vi "main.vi"() -> ()   [LabVIEW 2019]
uses:
  SubVI/ctl/335 state.ctl
  SubVI/ctl/Instrument Type.ctl
  SubVI/ctl/9T mag field stauts.ctl
  SubVI/ctl/warning.ctl
  SubVI/ctl/Gating type.ctl
  SubVI/ctl/Instrument.ctl
  <vilib>/NI/Modbus Library/API/Master/Modbus Master.lvclass
  SubVI/ctl/limit.ctl
  SubVI/ctl/set type.ctl
  SubVI/ctl/config.ctl
  SubVI/ctl/initialize.ctl
  <vilib>/NI/Modbus Library/API/Wrapper/Create TCP Master.vi
  lib/QDInstrument.dll
  SubVI/SubVI.lvlib
  SubVI/Add Seq.lvlib
  SubVI/User lib.lvlib
  <vilib>/NI/Modbus Library/API/Wrapper/API Main.lvlib
  SubVI/Get value.lvlib
  lib/Lake Shore 335/Lake Shore 335.lvlib
  SubVI/9T cmag.lvlib
  SubVI/nematic.lvlib
  lib/Lake Shore 325/Lake Shore 325.lvlib
  lib/Lake Shore 340/Lake Shore Cryotronics 340.lvlib
  SubVI/initialize.lvlib
panel:
  in  "gating type":T1
  out "?":string
  in  "行数":i32
  in  "是否处理":bool[](array[boolean])
  in  "层数":i32
  out "pzt volt":i32
  in  "warning":T2
  in  "Instrument Type":T3=enum."lengtou2"
  out "数据文件":path
  out "Aborting":bool
  in  "选项卡控件":T4(tab)=enum."335 2"
  out "Field":dbl
  out "Temperature":dbl
  in  "?":T5={"Field"=0.0, "Rate "=100.0, "Mode"=0, "Approach"=0, "field set"=FALSE} {"Approach" items=["Linear", "NoOvershoot", "Oscillate"]; "Mode" items=["Persistent", "Driven"]; "Rate" min=0.0 max=100.0; "Field" min=-140000.0 max=140000.0}
  in  "?":T6={"Temperature"=300.0, "Rate"=10.0, "Mode"=0, "temp set"=FALSE} {"Mode" items=["FastSettle", "NoOvershoot"]; "Rate" min=0.0 max=10.0; "Temperature" min=2.0 max=400.0}
  out "Status":i32(ring) items=["TemperatureUnknown"=0, "Stable"=1, "Tracking"=2, "Near"=5, "Chasing"=6, "Filling"=7, "Standby"=10, "Disabled"=13, "ImpedanceNotFunction"=14, "TempFailure"=15]
  out "Field Status":i32(ring) items=["MagnetUnknown"=0, "StablePersistent"=1, "WarmingSwitch"=2, "CoolingSwitch"=3, "StableDriven"=4, "Iterating"=5, "Charging"=6, "Discharging"=7, "CurrentError"=8, "MagnetFailure"=15]
  out "Chamber Status":i32(ring) items=["ChamberUnknown"=0, "PurgedAndSealed"=1, "VentedAndSealed"=2, "Sealed"=3, "Purging"=4, "Venting"=5, "PreHiVac"=6, "HighVac"=7, "PumpContinuous"=8, "VentContinuous"=9, "ChamberFailure"=15]
  in  "?":cluster{"chamber set":bool, "Code":i32} {"Code" items=["Seal", "PurgeAndSeal", "VentAndSeal", "PumpContinuous", "VentContinuous", "HighVacuum"]}
  out "Position":dbl
  in  "?":T7 {"Mode" items=["MoveToPosition", "MoveToLimitAndDefinePosition", "DefinePosition"]; "Speed" max=10}
  out "Rotate Temp":dbl
  in  "?":T8={"Temperature"=300.0, "Rate"=10.0, "temp set"=FALSE} {"Rate" min=0.0 max=10.0; "Temperature" min=2.0 max=400.0}
  in  "压缩机开启":bool
  in  "压缩机自动停机":bool=TRUE
  in  "自动控制":bool=TRUE
  out "325 Temp":dbl
  out "簇 2":T10 {"Heater Range" items=["Off", "Low (On)", "Medium", "High"]; "Heater Range 2" items=["Off", "Low (On)", "Medium", "High"]; "335 Status" items=["Unknow", "Stable", "Following Warm", "Following Cold", "Unfollowing"]}
  out "Out-plane angle":dbl
  in  "Position":T11
  in  "?":T12={"Field(Oe)"=0.0, "Approach"=enum."Linear", "Set Field"=FALSE, "Rate(Oe/s） "=30.0} {"Rate(Oe/s）" min=0.0 max=500.0; "Field(Oe)" min=-11000.0 max=11000.0}
  out "Field (Oe)":dbl
  out "Field Status":T13=enum."Stable"
  in  "335 2":T14={"Temperature"=300.0, "Rate (K/min)"=1.0, "Set Temp"=FALSE} {"Rate (K/min)" min=0.0 max=3.0; "Temperature" min=2.0 max=350.0}
  in  "压缩机启停":bool
  out "前面板":T15 {"340-A Status" items=["Unknow", "Stable", "Following Warm", "Following Cold", "Unfollowing"]; "Heater Range" items=["Off", "Low (On)", "High"]; "Heater Range 2" items=["Off", "Level 1", "Level 2", "Level 3", "Level 4", "Level 5"]; "340-B Status" items=["Unknow", "Stable", "Following Warm", "Following Cold", "Unfollowing"]}
  out "In-plane":dbl
  out "Out-plane":dbl
  in  "position":T16
  in  "?":T17={"Field(Oe)"=0.0, "Approach"=enum."Linear", "Field set"=FALSE, "Rate "=100.0} {"Rate" min=0.0 max=100.0; "Field(Oe)" min=-90000.0 max=90000.0}
  in  "?":T18={"Temperature"=300.0, "Rate"=10.0, "Temp set"=FALSE, "Ctrl On"=FALSE} {"Rate" min=0.0 max=10.0; "Temperature" min=2.0 max=400.0}
  in  "?":cluster{"Chamber set":bool, "Code":i32} {"Code" items=["Seal", "PurgeAndSeal", "VentAndSeal", "PumpContinuous", "VentContinuous", "HighVacuum"]}
  out "?":T19 {"Loop1 Output (%)" format="%.2f"; "Loop2 Output (%)" format="%.2f"}
  out "Temperature":dbl
  out "Temp Status":T9 items=["Unknow", "Stable", "Following Warm", "Following Cold", "Unfollowing"]
  out "Field (Oe)":dbl
  out "Field status":T13=enum."Stable"
  out "oscillating":bool=TRUE
  out "溢出？":bool
  out "错误输出 4":errorcluster caption="错误输出"
  out "错误输出 3":errorcluster caption="错误输出"
  out "错误输出 2":errorcluster caption="错误输出"
  out "错误输出":errorcluster
  out "psr saved":bool=TRUE
  out "seq":path
  in  "New psr":bool
  in  "Open":bool
  in  "Save as":bool
  in  "figure2datafile":path
  in  "figure1datafile":path
  in  "Save":bool
  in  "X 2":u16(ring)=1 items=["Timestamp(s)", "Time(s)", "TempB(K)", "TempA(K)", "Field(Oe)", "Position(degree)", "R1(Ohm)", "R1(V)", "R2(Ohm)", "R2(V)", "R3(Ohm)", "R3(V)", "R4(Ohm)", "R4(V)", "Source Current", "compliance(T1F0)", "Daul Gating chA Current(A)", "Daul Gating chA Current(V)", "Daul Gating chB Current(A)", "Daul Gating chB Voltage(V)", ""]
  out "XY图 2":cluster{"all rows":dbl[], "all rows":dbl[]}(graph) caption="XY图"
  in  "Y 2":u16(ring)=1 items=["Timestamp(s)", "Time(s)", "TempB(K)", "TempA(K)", "Field(Oe)", "Position(degree)", "R1(Ohm)", "R1(V)", "R2(Ohm)", "R2(V)", "R3(Ohm)", "R3(V)", "R4(Ohm)", "R4(V)", "Source Current", "compliance(T1F0)", "Daul Gating chA Current(A)", "Daul Gating chA Current(V)", "Daul Gating chB Current(A)", "Daul Gating chB Voltage(V)", ""]
  in  "Y":u16(ring)=1 items=["Timestamp(s)", "Time(s)", "Temp(K)", "Field(Oe)", "in plane position(degree)", "out plane position(degree)", "Rxx(Ohm)", "Ixx(A)", "Vxx(V)", "Ryx(Ohm)", "Iyx(A)", "Vyx(V)", "compliance(T1F0)", ""]
  out "Running":bool
  out "编辑列表框":bool=TRUE
  in  "Enable/Disable":bool
  in  "Delete":bool
  in  "Abort":bool
  out "XY图":cluster{"all rows":dbl[], "all rows":dbl[]}(graph)
  in  "X":u16(ring)=1 items=["Timestamp(s)", "Time(s)", "Temp(K)", "Field(Oe)", "in plane position(degree)", "out plane position(degree)", "Rxx(Ohm)", "Ixx(A)", "Vxx(V)", "Ryx(Ohm)", "Iyx(A)", "Vyx(V)", "compliance(T1F0)", ""]
  in  "树形":string(tree)
  in  "Run":bool
  in  "列表框":i32(listbox)=13
types:
  T1 = typedef "Gating type.ctl" = enum32{"null", "2614(daul)", "2400", "6517B"}
  T2 = typedef "warning.ctl" = cluster{"Compliance":bool}
  T3 = typedef "Instrument Type.ctl" = enum16{"PPMS", "VersaLab", "DynaCool", "SVSM", "PPMS-Rotate", "Lakeshore335", "lengtou2", "9T mag", "9T cmag rotate", "test"}
  T4 = enum32{"quantum design", "335", "335 2", "9T mag "}
  T5 = cluster{"Field":dbl, "Rate ":dbl, "Mode":i32, "Approach":i32, "field set":bool}
  T6 = cluster{"Temperature":dbl, "Rate":dbl, "Mode":i32, "temp set":bool}
  T7 = cluster{"position set":bool, "Position":dbl, "Speed":u16, "Mode":i32}
  T8 = cluster{"Temperature":dbl, "Rate":dbl, "temp set":bool}
  T9 = typedef "335 state.ctl" = u16
  T10 = cluster{"Output Value":dbl, "Heater Range":u16, "Ramping Active":bool, "Setpoint":dbl, "Temp B":dbl, "Temp A":dbl, "压缩机开启":bool, "335 Status":T9, "Ramping Active 2":bool, "Setpoint 2":dbl, "Output Value 2":dbl, "Heater Range 2":u16}
  T11 = cluster{"Postion":dbl, "Set Position ":bool, "Rate":dbl}
  T12 = cluster{"Field(Oe)":dbl, "Approach":enum16{"Linear", "Oscillate"}, "Set Field":bool, "Rate(Oe/s） ":dbl}
  T13 = typedef "9T mag field stauts.ctl" = enum16{"unknow", "Stable", "Sweep up", "Sweep down", "Sweep to zero", "Pause"}
  T14 = cluster{"Temperature":dbl, "Rate (K/min)":dbl, "Set Temp":bool}
  T15 = cluster{"Temp Sample":dbl, "Setpoint":dbl, "Heater Range":u16, "Output Value":dbl, "Ramping Active 340-B":bool, "340-B Status":T9, "Temp 2nd Stage":dbl, "Setpoint 2":dbl, "Heater Range 2":u16, "Output Value 2":dbl, "Ramping Active 340-A":bool, "340-A Status":T9, "压缩机开启":bool}
  T16 = cluster{"In plane":dbl, "Out plane":dbl, "Out-plane ":bool, "In-plane":bool}
  T17 = cluster{"Field(Oe)":dbl, "Approach":enum16{"Linear", "Oscillate"}, "Field set":bool, "Rate ":dbl}
  T18 = cluster{"Temperature":dbl, "Rate":dbl, "Temp set":bool, "Ctrl On":bool}
  T19 = cluster{"Temperature A":dbl, "Temperature B":dbl, "Temperature C":dbl, "Temperature D":dbl, "Loop1 Ramp?":bool, "Loop2 Ramp?":bool, "Loop1 Setpoint":dbl, "Loop2 Setpoint":dbl, "Output Pwr (%)":dbl, "Output Pwr (%)":dbl}
  T20 = typedef "Instrument.ctl" = cluster{"325 Resource ":refnum<visa-resource-name>, "Input (0:A) 325":u16, "Heater Output (1:1) 325":u16, "340 Resource":refnum<visa-resource-name>, "Input (0:A) 340":u16, "Loop (0: 1)":u16, "Input (0:B) 340":u16, "Loop (1: 1)":u16, "340 Status":refnum<vi>, "Instrument Type":T3, "quantum design":refnum<k24>, "semaphore 325":T21, "TCP master instance":refnum<class "Modbus Master.lvclass">, "M24C Resource":refnum<visa-resource-name>, "4G supply":refnum<visa-resource-name>, "Temp Status 24C":refnum<vi>, "Temp":refnum<vi>, "9T信号":T21, "limit":T22, "4g supply status":refnum<vi>, "vi路径":string, "in-plane":refnum<visa-resource-name>, "out-plane":refnum<visa-resource-name>, "in-plane signal":bool, "out-plane signal":bool, "in plane 信号":T21, "pzt volt":refnum<vi>, "Aborting":refnum<vi>, "数据文件":refnum<vi>, "warning":refnum<vi>, "750 visa":refnum<visa-resource-name>, "750 rotate":refnum<visa-resource-name>, "335 Status 2":refnum<vi>, "335 Resource ":refnum<visa-resource-name>, "Input (0:A) 335":u16, "Input (0:B) 335":u16, "Heater Output (1:1) 335":u16, "semaphore 340":T21, "semaphore 335":T21, "325 Status":refnum<vi>, "semaphore 750":T21, "750 field status":refnum<vi>, "camg 振荡状态":refnum<vi>, "列表框":refnum<vi>, "编辑列表框？":refnum<vi>, "camg Rate":refnum<vi>, "行数":refnum<vi>}
  T21 = typedef "Semaphore RefNum" = refnum<k1>
  T22 = typedef "limit.ctl" = cluster{"Field limit":dbl, "Field rate limit":dbl, "Temp limit":dbl, "Temp low limit":dbl, "Temp rate limit ":dbl}
  T23 = cluster{"Output Value":dbl, "Heater Range":u16, "Ramping Active":bool, "Setpoint":dbl, "Temp A":dbl, "Temp B":dbl, "压缩机开启":bool, T9, "Ramping Active 2":bool, "Setpoint 2":dbl, "Output Value 2":dbl, "Heater Range 2":u16}
  T24 = cluster{"Kelvin Reading":dbl, "Setpoint":dbl, "Heater Range":enum16{"Off", "1", "2", "3", "4", "5"}, "Heater Output":dbl, "Ramping Active/Inactive":bool, T9, "Kelvin Reading":dbl, "Setpoint":dbl, "Heater Range":enum16{"Off", "1", "2", "3", "4", "5"}, "Heater Output":dbl, "Ramping Active/Inactive":bool, T9, bool}
  T25 = typedef "set type.ctl" = enum16{"temp", "field", "position", "gating", "current", "time"}
  T26 = enum16{"open", "replace", "create", "open or create", "replace or create", "replace or create with confirmation"}
  T27 = typedef "config.ctl" = cluster{"initialize":T28, "6221":cluster{"6221 Resource":refnum<visa-resource-name>, "Delta status":bool, "电流|RMS(A)":dbl}, "SR830+6221":cluster{"source":u16, "Current(A)":dbl, "阻抗(Ohm)":dbl, "SR830 1":bool, "SR830 2":bool, "SR830 3":bool, "SR830 4":bool, "VISA 1":refnum<visa-resource-name>, "VISA 2":refnum<visa-resource-name>, "VISA 3":refnum<visa-resource-name>, "VISA 4":refnum<visa-resource-name>, "Reserve 1":i16, "Reserve 2":i16, "Reserve 3":i16, "Reserve 4":i16, "Sensitivity 1":i16, "Sensitivity 2":i16, "Sensitivity 3":i16, "Sensitivity 4":i16, "量程入 1":i32, "量程入 2":i32, "量程入 3":i32, "量程入 4":i32}, "2400":cluster{"2400":bool, "VISA":refnum<visa-resource-name>, "Output Level (0)":dbl, "Compliance  Level (0.1)":dbl}, "ch":cluster{"ch":i32[], "current":dbl[], "change?":bool[], "holding current\nwhen change ch?":bool}, "Instrument":T20, "2614B":cluster{"2614B chA":bool, "2614B chB":bool, "VISA":refnum<visa-resource-name>}, "33522b":cluster{"33522b resource name":refnum<visa-resource-name>, "零电压":dbl, "最大电压":dbl, "间隔":dbl, "最小电压":dbl, "PZT Scan?":bool}, "gating type":T1, "层数":i32, "行数":i32, "是否处理":bool[]}
  T28 = typedef "initialize.ctl" = enum16{"SR830", "keithley6221-SR830", "Delta", "Delta-tunnelling", "keithley6221-2182-DC", "PZT", "4200"}
  T29 = enum8{"Enabled", "Disabled", "Disabled and Grayed Out"}
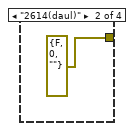
[diagram p2: hidden frame]
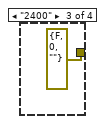
[diagram p3: hidden frame]
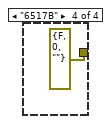
[diagram p4: hidden frame]
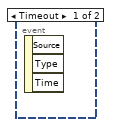
[diagram p6: hidden frame]
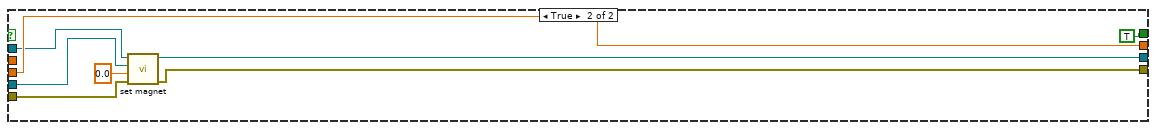
[diagram p7: hidden frame]
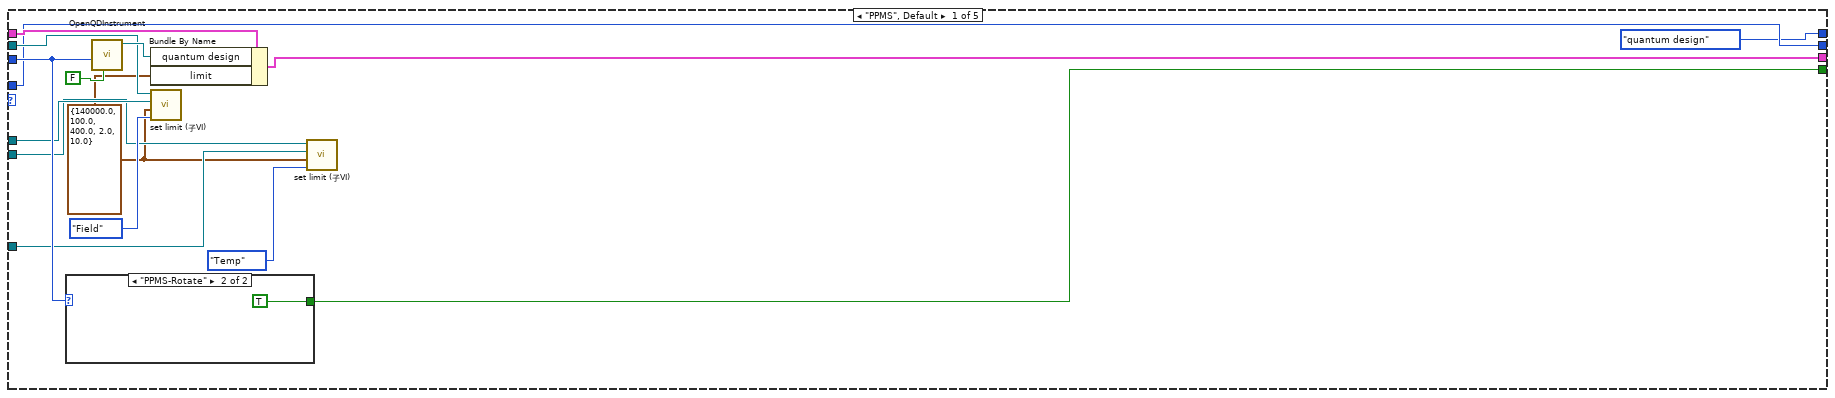
[diagram p9: hidden frame]
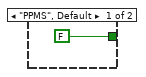
[diagram p10: hidden frame]
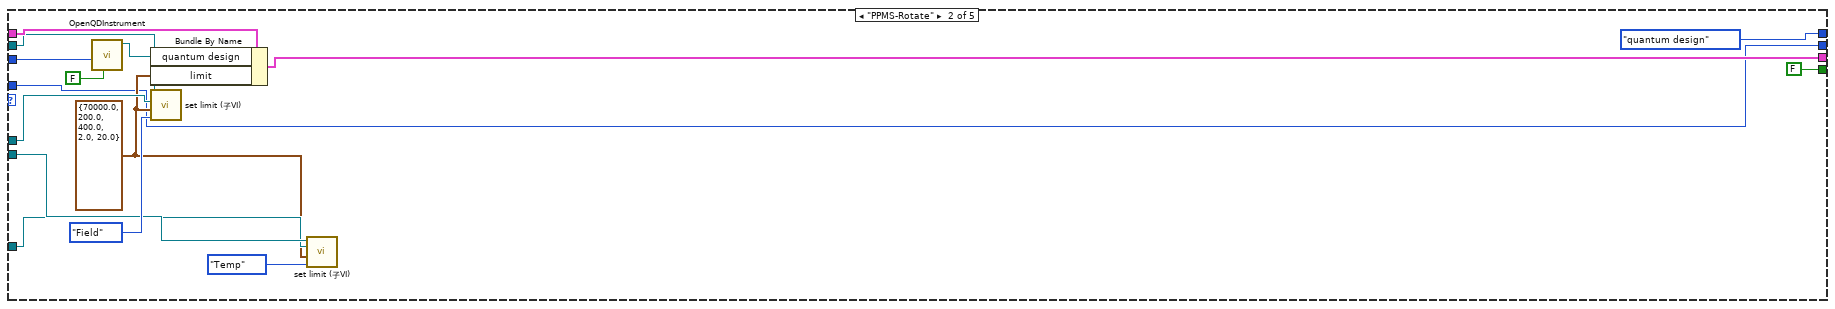
[diagram p11: hidden frame]
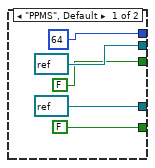
[diagram p13: hidden frame]
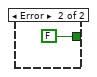
[diagram p14: hidden frame]
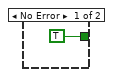
[diagram p15: hidden frame]
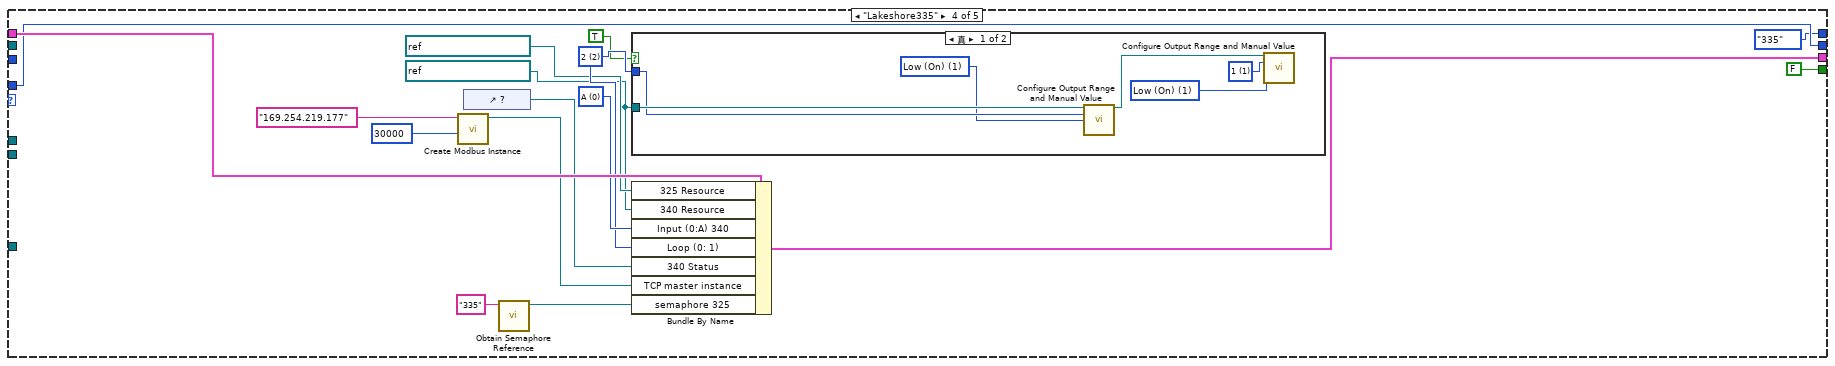
[diagram p18: hidden frame]
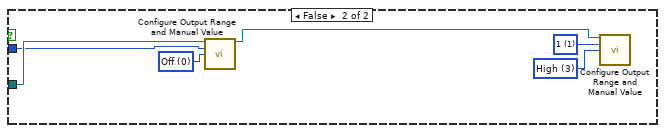
[diagram p19: hidden frame]
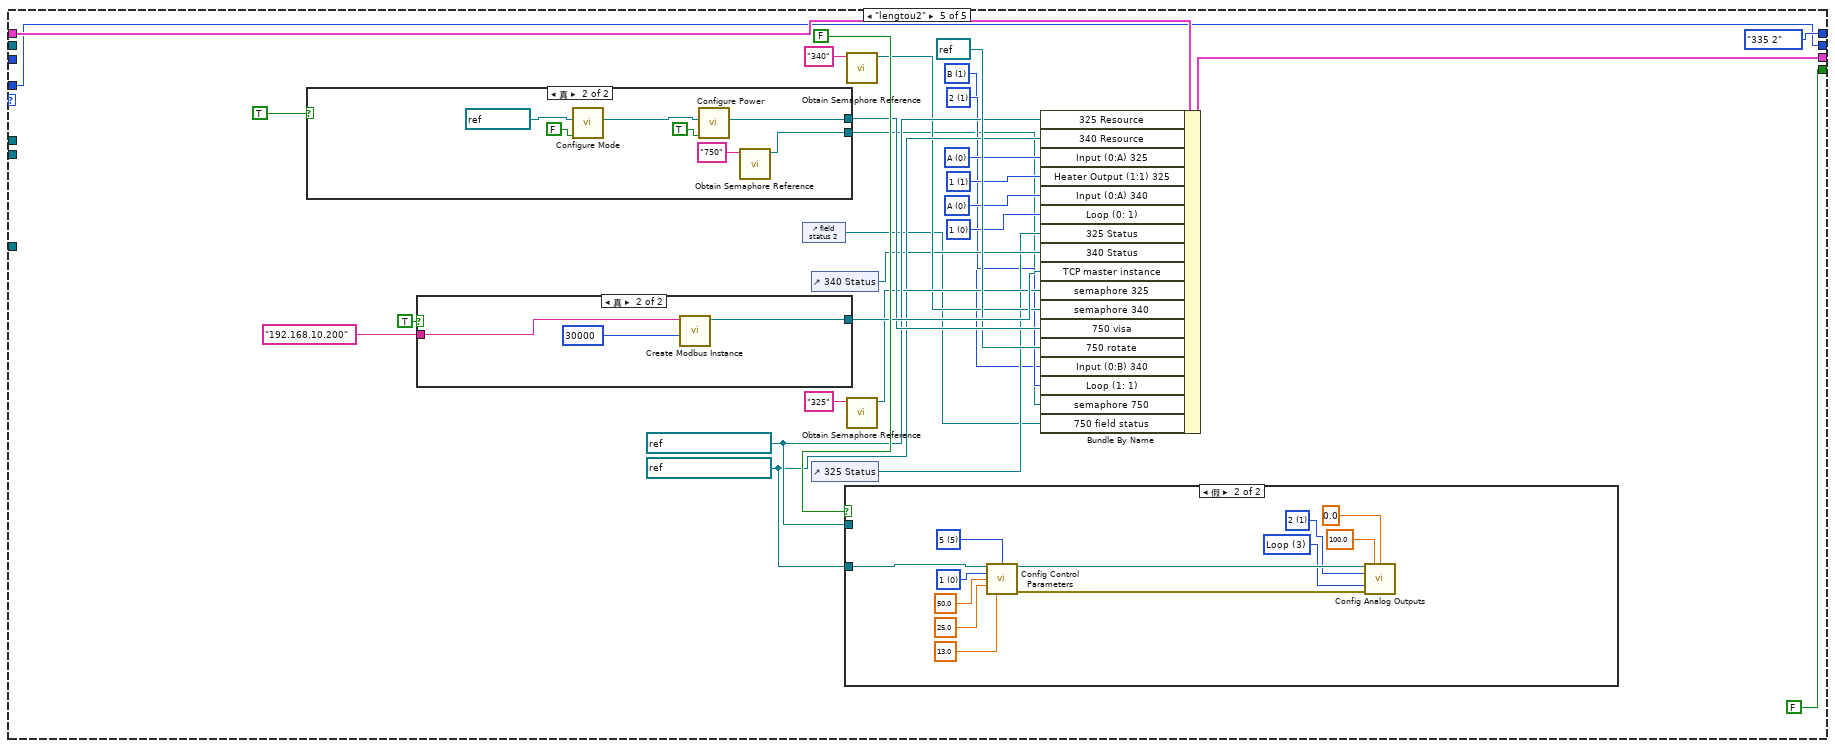
[diagram p20: hidden frame]
diagram:
  n1 = flat-sequence {
    tunnel: [w30] -> w1
    frame #0 {
      w32 = FALSE ("New psr")
      w33 = path "" ("添加的路径")
      n2 = case shown="真" FALSE {
        frame False {
        }
        frame True {
          w34 = FALSE ("x")
          n3 = flat-sequence {
            tunnel: w34 -> [w35]
            tunnel: w34 -> [w36]
            frame #0 {
              n4 = property class="Clust (严格)"("Visible"=w35) -> ()  [unwired: 2 in, 2 out]
              n5 = property class="Clust (严格)"("Visible"=w35) -> ()  [unwired: 2 in, 2 out]
              n6 = property on="Field" class="DigNum (严格)"("Visible"=w35) -> ()  [unwired: 2 in, 2 out]
              n7 = property on="Position" class="DigNum (严格)"("Visible"=w35) -> ()  [unwired: 2 in, 2 out]
              n8 = property class="Clust (严格)"("Visible"=w35) -> ()  [unwired: 2 in, 2 out]
              n9 = property on="Status" class="Ring (严格)"("Visible"=w35) -> ()  [unwired: 2 in, 2 out]
              n10 = property class="Clust (严格)"("Visible"=w35) -> ()  [unwired: 2 in, 2 out]
              n11 = property on="Field Status" class="Ring (严格)"("Visible"=w35) -> ()  [unwired: 2 in, 2 out]
              n12 = property on="Chamber Status" class="Ring (严格)"("Visible"=w35) -> ()  [unwired: 2 in, 2 out]
              n13 = property on="Temperature" class="DigNum (严格)"("Visible"=w35) -> ()  [unwired: 2 in, 2 out]
            }
            frame #1 {
              n14 = property class="Clust (严格)"("Visible"=w36) -> ()  [unwired: 2 in, 2 out]
              n15 = property on="自动控制" class="Bool (严格)"("Visible"=w36) -> ()  [unwired: 2 in, 2 out]
              n16 = property on="压缩机自动停机" class="Bool (严格)"("Visible"=w36) -> ()  [unwired: 2 in, 2 out]
              n17 = property on="压缩机开启" class="Bool (严格)"("Visible"=w36) -> ()  [unwired: 2 in, 2 out]
            }
          }
        }
      }
      n18 = property on="New psr" class="Bool (严格)"("Value"=w32) -> ()  [unwired: 2 in, 2 out]
      n19 = property on="Save as" class="Bool (严格)"("Value"=w32) -> ()  [unwired: 2 in, 2 out]
      n20 = property on="Save" class="Bool (严格)"("Value"=w32) -> ()  [unwired: 2 in, 2 out]
      n21 = property on="Open" class="Bool (严格)"("Value"=w32) -> ()  [unwired: 2 in, 2 out]
      n22 = property on="figure1datafile" class="Path"("Value"=w33) -> ()  [unwired: 2 in, 2 out]
      n23 = property on="figure2datafile" class="Path"("Value"=w33) -> ()  [unwired: 2 in, 2 out]
      n24 = property on="warning" class="Clust (严格)"("Value"=T2 {"Compliance"=FALSE} ("warning")) -> ()  [unwired: 2 in, 2 out]
      n25 = control-ref of="Temperature"() -> (w23:refnum<vi>)
      n26 = property on="选项卡控件" class="TabCtl (严格)"("BG Color"=u32 16448250 ("颜色:背景色")) -> ()  [unwired: 2 in, 2 out]
      n27 = control-ref of="Rate"() -> (w24:refnum<vi>)
      n28 = control-ref of="Field"() -> (w25:refnum<vi>)
      n29 = control-ref of="Rate"() -> (w22:refnum<vi>)
      n30 = case shown="\"9T mag\", \"9T cmag rotate\"" "Instrument Type" {
        selector: "Instrument Type" -> [_ _ w82 _ _]
        tunnel: "Instrument Type" -> [w46 w67 _ _ _]
        tunnel: T20 {"325 Resource "="", "Input (0:A) 325"=0, "Heater Output (1:1) 325"=0, "340 Resource"="", "Input (0:A) 340"=0, "Loop (0: 1)"=0, "Input (0:B) 340"=0, "Loop (1: 1)"=0, "340 Status"=refnum, "Instrument Type"=enum."PPMS", "quantum design"=refnum, "semaphore 325"=refnum, "TCP master instance"=refnum, "M24C Resource"="", "4G supply"="", "Temp Status 24C"=refnum, "Temp"=refnum, "9T信号"=refnum, "limit"={"Field limit"=0.0, "Field rate limit"=0.0, "Temp limit"=0.0, "Temp low limit"=0.0, "Temp rate limit "=0.0}, "4g supply status"=refnum, "vi路径"="", "in-plane"="", "out-plane"="", "in-plane signal"=FALSE, "out-plane signal"=FALSE, "in plane 信号"=refnum, "pzt volt"=refnum, "Aborting"=refnum, "数据文件"=refnum, "warning"=refnum, "750 visa"="", "750 rotate"="", "335 Status 2"=refnum, "335 Resource "="", "Input (0:A) 335"=0, "Input (0:B) 335"=0, "Heater Output (1:1) 335"=0, "semaphore 340"=refnum, "semaphore 335"=refnum, "325 Status"=refnum, "semaphore 750"=refnum, "750 field status"=refnum, "camg 振荡状态"=refnum, "列表框"=refnum, "编辑列表框？"=refnum, "camg Rate"=refnum, "行数"=refnum} ("Instrument") -> [w48 w64 w71 w151 w191]
        tunnel: [w49 w65 w97 w150 w190] -> w31
        tunnel: [w47 FALSE ("可见") FALSE ("可见") FALSE ("可见") FALSE ("可见")] -> w28
        tunnel: w25 -> [w45 w60 _ _ _]
        tunnel: w24 -> [w44 w59 _ _ _]
        tunnel: w23 -> [w42 w58 _ _ _]
        tunnel: w22 -> [w41 w57 _ _ _]
        tunnel: "Instrument Type" -> [w38 w55 _ w137 w164]
        tunnel: [w38 w55 Instrument_Type."9T mag" ("Instrument Type") w137 w164] -> w16
        tunnel: [enum32{"quantum design", "335", "9T mag "}."quantum design" ("选项卡控件 2") enum32{"quantum design", "335", "9T mag "}."quantum design" ("选项卡控件 2") T4."9T mag " ("选项卡控件") enum32{"quantum design", "335", "9T mag "}."335" ("选项卡控件 2") T4."335 2" ("选项卡控件")] -> w13
        frame "PPMS", Default {
          w40 = T22 {"Field limit"=140000.0, "Field rate limit"=100.0, "Temp limit"=400.0, "Temp low limit"=2.0, "Temp rate limit "=10.0} ("limit")
          n31 = case shown="\"PPMS-Rotate\"" w46 {
            tunnel: [FALSE ("可见") TRUE ("可见")] -> w47
            frame "PPMS", Default {
            }
            frame "PPMS-Rotate" {
            }
          }
          n32 = call "OpenQDInstrument.vi"("Remote"=FALSE, "Instrument Type"=w46) -> ("Instrument Ref"=w50:refnum<k24>)  [unwired: 6 in, 1 out]
          n33 = Bundle By Name(cluster=w48, "quantum design"=w50, "limit"=w40) -> (w49:T20)
          n34 = call "set limit (子VI).vi"("Temp or Field"=enum16{"Field", "Temp"}."Field", "limit"=w40, "rate"=w44, "value"=w45) -> ()  [unwired: 8 in]
          n35 = call "set limit (子VI).vi"("Temp or Field"=enum16{"Field", "Temp"}."Temp", "limit"=w40, "rate"=w41, "value"=w42) -> ()  [unwired: 8 in]
        }
        frame "PPMS-Rotate" {
          w56 = T22 {"Field limit"=70000.0, "Field rate limit"=200.0, "Temp limit"=400.0, "Temp low limit"=2.0, "Temp rate limit "=20.0} ("limit")
          n36 = call "OpenQDInstrument.vi"("Remote"=FALSE, "Instrument Type"=w67) -> ("Instrument Ref"=w66:refnum<k24>)  [unwired: 6 in, 1 out]
          n37 = Bundle By Name(cluster=w64, "quantum design"=w66, "limit"=w56) -> (w65:T20)
          n38 = call "set limit (子VI).vi"("Temp or Field"=enum16{"Field", "Temp"}."Field", "limit"=w56, "rate"=w59, "value"=w60) -> ()  [unwired: 8 in]
          n39 = call "set limit (子VI).vi"("Temp or Field"=enum16{"Field", "Temp"}."Temp", "limit"=w56, "rate"=w57, "value"=w58) -> ()  [unwired: 8 in]
        }
        frame "9T mag", "9T cmag rotate" {
          w76 = u8 1 items=["A", "B", "C", "D"] ("Input")
          n40 = case shown="\"9T cmag rotate\"" w82 {
            tunnel: [refnum<visa-resource-name> refnum ("VISA resource name out") w124] -> w88
            tunnel: [refnum<visa-resource-name> refnum ("VISA资源名称输出") w114] -> w87
            tunnel: [FALSE w117] -> w86
            tunnel: [FALSE w116] -> w85
            tunnel: [u8 64 ("y") u8 65 ("y")] -> w79
            frame "PPMS", Default {
            }
            frame "9T cmag rotate" {
              n41 = call "PZT init.vi"("Ch"=enum16{"CH1", "CH2", "CH3"}."CH1", "Communication"=enum16{"USB", "LAN"}."USB", "VISA resource name"=refnum<visa-resource-name> "COM12" ("in-plane")) -> ("错误输出"=w119:errorcluster, "VISA资源名称输出"=w114:refnum<visa-resource-name>)  [unwired: 1 in]
              n42 = call "Initialize.vi"("VISA resource name in"=refnum<visa-resource-name> "COM13" ("out-plane")) -> ("error out"=w118:errorcluster, "VISA resource name out"=w124:refnum<visa-resource-name>)  [unwired: 9 in]
              n43 = case shown="错误 .." w119 {
                tunnel: [TRUE FALSE] -> w117
                frame No Error {
                }
                frame Error {
                }
              }
              n44 = case shown="无错误" w118 {
                tunnel: [TRUE FALSE] -> w116
                frame No Error {
                }
                frame Error {
                }
              }
            }
          }
          n45 = call "CC_Initialize.vi"("Serial Configuration"=cluster{"Baud Rate":u32} {"Baud Rate"=9600}, "VISA resource name"=refnum<visa-resource-name> "COM3" ("335 Resource")) -> ("VISA resource name out"=w100:refnum<visa-resource-name>)  [unwired: 8 in, 1 out]
          n46 = call "24C get control.vi"("VISA In"=w100) -> ("Control?"=w96:bool, "VISA out"=w78:refnum<visa-resource-name>)  [unwired: 7 in, 1 out]
          n47 = case shown="假" w96 {
            frame False {
              n48 = flat-sequence {
                frame #0 {
                  n49 = One Button Dialog(message="M24C未处于控制状态，请检查" ("消息")) -> ()  [unwired: 1 in, 1 out]
                }
                frame #1 {
                  n50 = Stop(stop? (T)=FALSE ("停止？(T)")) -> ()
                }
              }
            }
            frame True {
            }
          }
          n51 = call "Input_Get_Config.vi"("VISA In"=w78, "Input"=w76) -> ("Sensor Index"=w81:u8, "VISA Out"=w77:refnum<visa-resource-name>)  [unwired: 5 in, 3 out]
          n52 = Equal?(x=w81, y=w79) -> (x = y?=w80:bool)
          n53 = case shown="假" w80 {
            tunnel: w79 -> [w104 _]
            tunnel: w77 -> [w107 w108]
            tunnel: [w105 w108] -> w75
            frame False {
              w106 = u8 1 items=["A", "B", "C", "D"] ("Input")
              n54 = call "Input_SensorTypeIndex.vi"("VISA in"=w107, "Input"=w106, "Sensor"=w104) -> ("VISA out"=w105:refnum<visa-resource-name>)  [unwired: 2 in, 2 out]
            }
            frame True {
            }
          }
          n55 = case shown="真" TRUE {
            tunnel: refnum<visa-resource-name> "GPIB0::1::INSTR" ("VISA Resource Name") -> [w129 w133]
            tunnel: [w129 w131] -> w98
            frame False {
            }
            frame True {
              n56 = call "4G Initialize.vi"("Reset (T: Reset)"=TRUE, "ID Query (T: Check)"=FALSE, "VISA Resource Name"=w133) -> ("VISA Resource Out"=w131:refnum<visa-resource-name>)  [unwired: 3 in, 1 out]
            }
          }
          n57 = control-ref of="Temperature"() -> (w94:refnum<vi>)
          n58 = control-ref of="Temp Status"() -> (w95:refnum<vi>)
          n59 = control-ref of="field status"() -> (w91:refnum<vi>)
          n60 = control-ref of="335 Status"() -> (w69:refnum<vi>)
          n61 = control-ref of="pzt volt"() -> (w73:refnum<vi>)
          n62 = call <vilib>:"Obtain Semaphore Reference.vi"("name (unnamed)"="9T mag") -> ("semaphore"=w92:T21)  [unwired: 4 in, 2 out]
          n63 = call <vilib>:"Obtain Semaphore Reference.vi"("name (unnamed)"="in plane") -> ("semaphore"=w83:T21)  [unwired: 4 in, 2 out]
          n64 = Bundle By Name(cluster=w71, "M24C Resource"=w75, "4G supply"=w98, "Temp Status 24C"=w95, "4g supply status"=w91, "Temp"=w94, "9T信号"=w92, "limit"=T22 {"Field limit"=90000.0, "Field rate limit"=100.0, "Temp limit"=325.0, "Temp low limit"=1.6, "Temp rate limit "=10.0}, "in-plane"=w87, "out-plane"=w88, "in-plane signal"=w86, "out-plane signal"=w85, "in plane 信号"=w83, "pzt volt"=w73, "335 Status 2"=w69) -> (w97:T20)
          "pzt volt" <- 0 ("pzt volt")
        }
        frame "Lakeshore335" {
          w143 = u16 2 items=["1"=1, "2"=2] ("Heater Output (1:1)")
          w149 = u16 0 items=["A", "B"] ("Input (0:A)")
          w139 = refnum<visa-resource-name> "GPIB0::12::INSTR" ("335 Resource")
          n65 = call-poly <vilib>:"Create Modbus Instance.vi"("connect timeout ms"=30000, "address"="169.254.219.177") -> ("TCP master instance"=w138:refnum<class "Modbus Master.lvclass">)  [unwired: 8 in, 1 out]
          n66 = control-ref of="?"() -> (w140:refnum<vi>)
          n67 = call <vilib>:"Obtain Semaphore Reference.vi"("name (unnamed)"="335") -> ("semaphore"=w146:T21)  [unwired: 4 in, 2 out]
          n68 = case shown="真" TRUE {
            tunnel: w139 -> [w157 w163]
            tunnel: w143 -> [w156 w162]
            frame True {
              w152 = u16 1 items=["1"=1, "2"=2] ("Heater Output (1:1)")
              w153 = u16 1 items=["Off", "Low (On)", "Medium", "High"] ("Range (0:Off)")
              w155 = u16 1 items=["Off", "Low (On)", "Medium", "High"] ("Range (0:Off)")
              n69 = call "Configure Output Range and Manual Value.vi"("VISA resource name"=w157, "Heater Output (1:1)"=w156, "Range (0:Off)"=w155) -> ("VISA resource name out"=w154:refnum<visa-resource-name>)  [unwired: 11 in, 1 out]
              n70 = call "Configure Output Range and Manual Value.vi"("VISA resource name"=w154, "Heater Output (1:1)"=w152, "Range (0:Off)"=w153) -> ()  [unwired: 11 in, 2 out]
            }
            frame False {
              w159 = u16 3 items=["Off", "Low (On)", "Medium", "High"] ("Range (0:Off)")
              w160 = u16 1 items=["1"=1, "2"=2] ("Heater Output (1:1)")
              w161 = u16 0 items=["Off", "Low (On)", "Medium", "High"] ("Range (0:Off)")
              n71 = call "Configure Output Range and Manual Value.vi"("VISA resource name"=w163, "Heater Output (1:1)"=w162, "Range (0:Off)"=w161) -> ("VISA resource name out"=w158:refnum<visa-resource-name>)  [unwired: 11 in, 1 out]
              n72 = call "Configure Output Range and Manual Value.vi"("VISA resource name"=w158, "Heater Output (1:1)"=w160, "Range (0:Off)"=w159) -> ()  [unwired: 11 in, 2 out]
            }
          }
          n73 = Bundle By Name(cluster=w151, "325 Resource"=refnum<visa-resource-name> "GPIB0::13::INSTR", "340 Resource"=w139, "Input (0:A) 340"=w149, "Loop (0: 1)"=w143, "340 Status"=w140, "TCP master instance"=w138, "semaphore 325"=w146) -> (w150:T20)
        }
        frame "lengtou2" {
          w167 = u16 1 items=["A", "B", "C", "D"] ("Input (0: A)")
          w168 = u16 1 items=["1", "2"] ("Loop (0: 1)")
          w169 = u16 0 items=["A", "B", "C", "D"] ("Input (0: A)")
          w170 = u16 0 items=["1", "2"] ("Loop (0: 1)")
          w180 = refnum<visa-resource-name> "GPIB0::13::INSTR" ("325 Resource")
          w173 = u16 1 items=["1"=1, "2"=2] ("Heater Output (1:1)")
          w174 = u16 0 items=["A", "B"] ("Input (0:A)")
          w177 = refnum<visa-resource-name> "GPIB0::14::INSTR" ("335 Resource")
          n74 = case shown="真" TRUE {
            tunnel: [refnum<visa-resource-name> refnum ("VISA resource name out") w201] -> w184
            tunnel: [w196 w198] -> w166
            frame False {
              w196 = T21 refnum items=["semaphore"] ("semaphore")
            }
            frame True {
              n75 = call "Configure Mode.vi"("Mode? (T: CURR)"=FALSE, "VISA resource name"=refnum<visa-resource-name> "COM4") -> ("VISA resource name out"=w203:refnum<visa-resource-name>)  [unwired: 8 in, 1 out]
              n76 = call "Configure Power.vi"("Power ON? (T: ON)"=TRUE, "VISA resource name"=w203) -> ("VISA resource name out"=w201:refnum<visa-resource-name>)  [unwired: 8 in, 1 out]
              n77 = call <vilib>:"Obtain Semaphore Reference.vi"("name (unnamed)"="750") -> ("semaphore"=w198:T21)  [unwired: 4 in, 2 out]
            }
          }
          n78 = case shown="真" TRUE {
            tunnel: "192.168.10.200" ("address") -> [_ w195]
            tunnel: [refnum<class "Modbus Master.lvclass"> refnum ("TCP master instance") w193] -> w185
            frame False {
            }
            frame True {
              n79 = call-poly <vilib>:"Create Modbus Instance.vi"("connect timeout ms"=30000, "address"=w195) -> ("TCP master instance"=w193:refnum<class "Modbus Master.lvclass">)  [unwired: 8 in, 1 out]
            }
          }
          n80 = control-ref of="field status 2"() -> (w165:refnum<vi>)
          n81 = control-ref of="340 Status"() -> (w172:refnum<vi>)
          n82 = control-ref of="325 Status"() -> (w171:refnum<vi>)
          n83 = case shown="假" FALSE {
            tunnel: w180 -> [w214 _]
            tunnel: w177 -> [w210 w221]
            frame True {
              w209 = u16 5 items=["Off", "1", "2", "3", "4", "5"] ("Heater Range (0: Off)")
              w208 = u16 0 items=["1", "2"] ("Loop (0: 1)")
              w211 = u16 2 items=["25 Ohm"=1, "50 Ohm"=2] ("Heater Resistance (1:25 Ohm)")
              w212 = u16 1 items=["Off", "Low (loop 1) or On (loop 2)", "High (loop 1)"] ("Heater Range (0:Off)")
              w213 = u16 1 items=["Loop 1"=1, "Loop 2"=2] ("Loop (1:Loop 1)")
              n84 = call "Config Control Parameters.vi"("VISA resource name"=w210, "Heater Range (0: Off)"=w209, "Loop (0: 1)"=w208, "Gain (P) (0.0)"=50.0, "Reset (I) (0.0)"=25.0, "Rate (D) (0)"=13.0) -> ()  [unwired: 8 in, 2 out]
              n85 = call "Configure Control Parameters.vi"("VISA resource name"=w214, "Loop (1:Loop 1)"=w213, "Heater Range (0:Off)"=w212, "Heater Resistance (1:25 Ohm)"=w211) -> ()  [unwired: 10 in, 2 out]
            }
            frame False {
              w215 = u16 3 items=["Off", "Input", "Manual", "Loop"] ("Analog Output\nMode (0: Off)")
              w218 = u16 1 items=["1", "2"] ("Loop (0: 1)")
              w226 = u16 5 items=["Off", "1", "2", "3", "4", "5"] ("Heater Range (0: Off)")
              w225 = u16 0 items=["1", "2"] ("Loop (0: 1)")
              n86 = call "Config Control Parameters.vi"("VISA resource name"=w221, "Heater Range (0: Off)"=w226, "Loop (0: 1)"=w225, "Gain (P) (0.0)"=50.0, "Reset (I) (0.0)"=25.0, "Rate (D) (0)"=13.0) -> ("VISA resource name out"=w220:refnum<visa-resource-name>, "error out"=w219:errorcluster)  [unwired: 8 in]
              n87 = call "Config Analog Outputs.vi"("VISA resource name"=w220, "High Value (0.0000)"=100.0, "Low Value (0.0000)"=0.0, "Analog Output (0: 1)"=w218, "Analog Output\nMode (0: Off)"=w215, "error in (no error)"=w219) -> ()  [unwired: 8 in, 2 out]
            }
          }
          n88 = call <vilib>:"Obtain Semaphore Reference.vi"("name (unnamed)"="340") -> ("semaphore"=w175:T21)  [unwired: 4 in, 2 out]
          n89 = call <vilib>:"Obtain Semaphore Reference.vi"("name (unnamed)"="325") -> ("semaphore"=w178:T21)  [unwired: 4 in, 2 out]
          n90 = Bundle By Name(cluster=w191, "325 Resource"=w180, "340 Resource"=w177, "Input (0:A) 325"=w174, "Heater Output (1:1) 325"=w173, "Input (0:A) 340"=w169, "Loop (0: 1)"=w170, "325 Status"=w171, "340 Status"=w172, "TCP master instance"=w185, "semaphore 325"=w178, "semaphore 340"=w175, "750 visa"=w184, "750 rotate"=refnum<visa-resource-name> refnum, "Input (0:B) 340"=w167, "Loop (1: 1)"=w168, "semaphore 750"=w166, "750 field status"=w165) -> (w190:T20)
        }
      }
      n91 = control-ref of="行数"() -> (w7:refnum<vi>)
      n92 = Current VI's Path() -> (path=w19:path)
      n93 = control-ref of="编辑列表框"() -> (w10:refnum<vi>)
      n94 = control-ref of="oscillating"() -> (w12:refnum<vi>)
      n95 = control-ref of="数据文件"() -> (w15:refnum<vi>)
      n96 = Strip Path(path=w19) -> (stripped path=w20:path)  [unwired: 1 out]
      n97 = control-ref of="warning"() -> (w14:refnum<vi>)
      n98 = Path To String(path=w20) -> (string=w18:string)
      n99 = property on="选项卡控件" class="TabCtl (严格)"("Value"=w13) -> ()  [unwired: 2 in, 2 out]
      n100 = property on="Rotate Temp" class="DigNum (严格)"("Visible"=w28) -> ()  [unwired: 2 in, 2 out]
      n101 = control-ref of="列表框"() -> (w11:refnum<vi>)
      n102 = control-ref of="Aborting"() -> ()  [unwired: 1 out]
      n103 = control-ref of="Rate"() -> (w9:refnum<vi>)
      n104 = control-ref of="Abort"() -> (w8:refnum<vi>)
      n105 = Bundle By Name(cluster=w31, "Instrument Type"=w16, "vi路径"=w18, "Aborting"=w8, "数据文件"=w15, "warning"=w14, "camg 振荡状态"=w12, "列表框"=w11, "编辑列表框？"=w10, "camg Rate"=w9, "行数"=w7) -> (w30:T20)
      "oscillating" <- FALSE ("oscillating")
    }
  }
  n106 = call "log save.vi"("Instrument"=w1) -> ()  [unwired: 11 in]
  n107 = while {
    tunnel: w1 -> [_]
    stop <- FALSE stop-if-true
    n108 = Wait Until Next ms Multiple(millisecond multiple=u32 5000 ("毫秒倍数")) -> ()  [unwired: 1 out]
    n109 = Unbundle By Name("warning") -> ("Compliance"=w230:bool)
    n110 = case shown="真" w230 {
      tunnel: "warning" -> [_ w233]
      frame False {
      }
      frame True {
        n111 = Bundle By Name(cluster=w233, "Compliance"=FALSE) -> (w231:T2)
        n112 = property on="warning" class="Clust (严格)"("Value"=w231) -> ()  [unwired: 2 in, 2 out]
        n113 = One Button Dialog(message="在之前的测量中，有一段时间，6221达到了compliance，请注意检查数据" ("消息")) -> ()  [unwired: 1 in, 1 out]
      }
    }
  }
  n114 = while {
    shift-right: [w236] -> _
    shift-left: 0 -> [w245]
    shift-right: [w258] -> _
    shift-left: 0 -> [w259]
    tunnel: w1 -> [w255]
    shift-right: [w237] -> _
    shift-left: path "" ("figure1datafile") -> [w242]
    shift-right: [w256] -> _
    shift-left: path "" ("figure2datafile") -> [w257]
    i -> [w252]
    stop <- FALSE stop-if-true
    n115 = Unbundle By Name(w255) -> ("Instrument Type"=w254:T3)
    n116 = Wait (ms)(milliseconds to wait=u32 300 ("等待时间（毫秒）")) -> ()  [unwired: 1 out]
    n117 = case shown="\"9T mag\"" w254 {
      selector: w254 -> [_ _ _ w303]
      tunnel: w255 -> [w273 w276 w288 w305]
      tunnel: w252 -> [w272 _ _ _]
      frame "Lakeshore335" {
        n118 = call "335 Read and Compressor auto control(SubVI).vi"("压缩机自动停机"="压缩机自动停机", "自动控制"="自动控制", "数值"=w272, "Instrument"=w273) -> ("325 Temp"=→"325 Temp":dbl, "簇"=→"簇 2":T23)  [unwired: 6 in]
      }
      frame "lengtou2" {
        n119 = call "340 Read and Compressor auto control(SubVI).vi"("Instrument"=w276) -> ("Output Field (Gs)"=→"Field (Oe)":dbl, "output"=→"前面板":T24, "field status 2"=→"Field Status":T13)  [unwired: 8 in]
      }
      frame "9T mag" {
        n120 = Unbundle By Name(w288) -> ("4G supply"=w287:refnum<visa-resource-name>)
        n121 = call "24C and 4G Read (SubVI).vi"("Instrument"=w288) -> ("field status"=→"Field status":T13, "field(Oe)"=w281:dbl, "输出簇"=w292:T19, "下拉列表"=→"Temp Status":T9, "out-plane position"=→"Out-plane":dbl, "in-plane position"=→"In-plane":dbl)  [unwired: 5 in]
        "?" <- w292
        "Field (Oe)" <- w281
        n122 = Absolute Value(x=w281) -> (abs(x)=w280:dbl)
        n123 = Unbundle(w292) -> ("Temperature B"=w285:dbl, "Temperature D"=w284:dbl)  [unwired: 8 out]
        "Temperature" <- w285
        n124 = call "warning display.vi"("TempD(K) 2"=w284, "TempB(K) 2"=w285, "Field(Oe) 2"=w281) -> ()  [unwired: 9 in]
        n125 = Greater?(x=w280, y=0.0) -> (0:w282:bool)
        n126 = Greater?(x=w284, y=4.6) -> (0:w286:bool)
        n127 = case shown="真" w282 {
          tunnel: w287 -> [_ w294]
          tunnel: w286 -> [_ w293]
          frame False {
          }
          frame True {
            n128 = case shown="真" w293 {
              tunnel: w294 -> [_ w297]
              tunnel: w293 -> [_ _]
              frame False {
              }
              frame True {
                n129 = flat-sequence {
                  tunnel: w297 -> [w302]
                  frame #0 {
                    n130 = call "4G Write.vi"("write buffer (\"\")"="SWEEP PAUSE " ("write buffer (\"\")"), "VISA session"=w302) -> ()  [unwired: 1 in, 3 out]
                  }
                }
                n131 = property on="Running" class="Bool (严格)"() -> ("Value"=w296:bool)  [unwired: 2 in, 2 out]
                n132 = case shown="真" w296 {
                  tunnel: ["TempD温度过高，磁场已暂停" ("message") "TempD温度过高，seq已终止，磁场已暂停" ("message")] -> w295
                  frame False {
                  }
                  frame True {
                    n133 = property on="Abort" class="Bool (严格)"("Val(Sgnl)"=TRUE ("Value (Signaling)")) -> ()  [unwired: 2 in, 2 out]
                  }
                }
                n134 = One Button Dialog(message=w295) -> ()  [unwired: 1 in, 1 out]
              }
            }
          }
        }
      }
      frame "PPMS", Default {
        n135 = Unbundle By Name(w305) -> ("quantum design"=w304:refnum<k24>)
        n136 = case shown="\"Lakeshore335\"" w303 {
          tunnel: [0.0 ("Result") w315] -> w306
          tunnel: w304 -> [_ w314]
          frame "PPMS", Default {
          }
          frame "Lakeshore335" {
            n137 = call "Get Rotate Temp(SubVI).vi"(".NET引用句柄输入"=w314) -> ("Result"=w315:dbl)  [unwired: 10 in]
          }
        }
        "Rotate Temp" <- w306
        n138 = call "get poisition.vi"("Instrument Ref In"=w304) -> ("Position"=→"Position":dbl)  [unwired: 4 in, 2 out]
        n139 = call "GetChamber.vi"("Instrument Ref In"=w304) -> ("Chamber\nStatus"=→"Chamber Status":i32)  [unwired: 3 in, 3 out]
        n140 = call "GetField.vi"("Instrument Ref In"=w304) -> ("Field\nStatus"=→"Field Status":i32, "Field"=→"Field":dbl)  [unwired: 4 in, 3 out]
        n141 = call "GetTemperature.vi"("Instrument Ref In"=w304) -> ("Temperature\nStatus"=→"Status":i32, "Temperature"=→"Temperature":dbl)  [unwired: 4 in, 3 out]
      }
    }
    n142 = event shown="[0] 超时" {
      selector: _ -> [_ _]
      dyn-events: _ -> [_ _]
      timeout: 200 -> [_ _]
      tunnel: [FALSE TRUE] -> w248
      event Timeout {
        n143 = event-data() -> ()  [unwired: 1 in, 3 out]
      }
      event "Y 2", "X 2": Value Change {
        n144 = event-data() -> ()  [unwired: 1 in, 6 out]
      }
    }
    n145 = event shown="[0] 超时" {
      selector: _ -> [_ _]
      dyn-events: _ -> [_ _]
      timeout: 200 -> [_ _]
      tunnel: [FALSE w265] -> _
      tunnel: [_ w265] -> w246
      event Timeout {
        n146 = event-data() -> ()  [unwired: 1 in, 3 out]
      }
      event "Y", "X": Value Change {
        w265 = TRUE
        n147 = event-data() -> ()  [unwired: 1 in, 6 out]
      }
    }
    n148 = Path To String(path="figure2datafile") -> (string=w261:string)
    n149 = Path To String(path="figure1datafile") -> (string=w262:string)
    n150 = String Length(string=w261) -> (length=w244:i32)
    n151 = String Length(string=w262) -> (length=w238:i32)
    n152 = control-ref of="Y 2"() -> (w251:refnum<vi>)
    n153 = control-ref of="X 2"() -> (w250:refnum<vi>)
    n154 = control-ref of="Y"() -> (w241:refnum<vi>)
    n155 = control-ref of="X"() -> (w240:refnum<vi>)
    n156 = control-ref of="XY图 2"() -> (w249:refnum<vi>)
    n157 = call "show figure (SubVI).vi"("y"=w248, "XYGraph引用句柄"=w249, "文件名长度"=w244, "上次的数据列数"=w259, "新数据文件"="figure2datafile", "Y输入"=w251, "X输入"=w250, "上一次的数据文件"=w257) -> ("figure2datafile输出"=w256:path, "数值输出"=w258:i32)  [unwired: 6 in]
    n158 = control-ref of="XY图"() -> (w239:refnum<vi>)
    n159 = call "show figure (SubVI).vi"("y"=w246, "XYGraph引用句柄"=w239, "文件名长度"=w238, "上次的数据列数"=w245, "新数据文件"="figure1datafile", "Y输入"=w241, "X输入"=w240, "上一次的数据文件"=w242) -> ("figure2datafile输出"=w237:path, "数值输出"=w236:i32)  [unwired: 6 in]
  }
  n160 = while {
    tunnel: w1 -> [w318]
    stop <- FALSE stop-if-true
    n161 = Unbundle By Name(w318) -> ("4G supply"=w317:refnum<visa-resource-name>, "9T信号"=w316:T21)  [unwired: 2 out]
    n162 = event shown="[1] \"oscillating\": 值改变" {
      selector: _ -> [_ _]
      dyn-events: _ -> [_ _]
      timeout: _ -> [_ _]
      tunnel: w317 -> [_ w323]
      tunnel: w316 -> [_ w322]
      event Timeout {
        n163 = event-data() -> ()  [unwired: 1 in, 3 out]
      }
      event "oscillating": Value Change {
        n164 = event-data() -> ()  [unwired: 1 in, 6 out]
        n165 = property on="Rate" class="DigNum (严格)"() -> ("Value"=w321:dbl)  [unwired: 2 in, 2 out]
        n166 = stacked-sequence {
          tunnel: [w336] -> _
          tunnel: [w337] -> _
          tunnel: errorcluster {"status"=FALSE, "code"=0, "source"=""} ("错误输入（无错误）") -> [w338]
          tunnel: w321 -> [w332]
          tunnel: w322 -> [w330]
          tunnel: w323 -> [w341]
          tunnel: [w331] -> w320
          frame #0 {
            n167 = flat-sequence {
              tunnel: w330 -> [w345]
              tunnel: w338 -> [w346]
              tunnel: w341 -> [w347]
              tunnel: [w347] -> w329
              tunnel: [w346] -> w328
              tunnel: [w344] -> w327
              tunnel: [w352] -> w343
              tunnel: [w350] -> w339
              tunnel: w329 -> [w351]
              tunnel: w328 -> [w349]
              tunnel: [w348] -> w326
              tunnel: w327 -> [w348]
              frame #0 {
                n168 = call <vilib>:"Acquire Semaphore.vi"("semaphore"=w345) -> ("semaphore out"=w344:T21)  [unwired: 4 in, 2 out]
              }
              frame #1 {
                n169 = call "4G Read Mag Current.vi"("error in (no error)"=w349, "VISA session"=w351) -> ("error out"=w350:errorcluster, "response out"=w352:string)  [unwired: 1 in, 1 out]
              }
            }
            n170 = call <vilib>:"Release Semaphore.vi"("semaphore"=w326) -> ("semaphore out"=w325:T21)  [unwired: 5 in, 1 out]
            n171 = Match Pattern(string=w343, regular expression=" " ("正则表达式")) -> (before substring=w340:string)  [unwired: 1 in, 3 out]
            n172 = Fract/Exp String To Number(string=w340) -> (number=w335:dbl)  [unwired: 3 in, 1 out]
            n173 = Multiply(x=w335, y=1000.0) -> (x*y=w334:dbl)
            n174 = while {
              shift-right: [w365] -> _
              shift-left: w334 -> [w360]
              tunnel: w341 -> [w366]
              tunnel: w339 -> [w364]
              tunnel: [w363] -> w336
              tunnel: [w362] -> w337
              tunnel: w325 -> [w361]
              tunnel: w332 -> [w358]
              tunnel: [FALSE ("oscillating")] -> w331
              stop <- w355 stop-if-true
              n175 = Absolute Value(x=w360) -> (abs(x)=w359:dbl)
              n176 = Less?(x=w359, y=50.0) -> (x < y?=w367:bool)
              n177 = case shown="假" w367 {
                tunnel: [FALSE TRUE] -> w356
                tunnel: w366 -> [w381 w413]
                tunnel: w360 -> [w379 w414]
                tunnel: [w372 w414] -> w365
                tunnel: w364 -> [w377 w411]
                tunnel: [w375 w410] -> w363
                tunnel: [w374 w409] -> w362
                tunnel: w361 -> [w370 w408]
                tunnel: w358 -> [w371 _]
                frame False {
                  n178 = Multiply(x=w379, y=-0.7) -> (x*y=w373:dbl)
                  n179 = Round To Nearest(number=w373) -> (nearest integer value=w372:dbl)
                  n180 = call "set magnet.vi"("Rate(Oe/s)"=w371, "error in (no error)"=w377, "Magnet field(Oe)"=w372, "semaphore"=w370, "VISA Resource Name"=w381) -> ("error out"=w376:errorcluster, "semaphore out"=w369:T21, "dup VISA session"=w378:refnum<visa-resource-name>)  [unwired: 4 in]
                  n181 = while {
                    tunnel: w378 -> [w400]
                    tunnel: w376 -> [w399]
                    tunnel: [w397] -> w375
                    tunnel: [w398] -> w374
                    tunnel: w369 -> [w395]
                    tunnel: w372 -> [w387]
                    stop <- w385 stop-if-true
                    n182 = call <vilib>:"Acquire Semaphore.vi"("semaphore"=w395) -> ("semaphore out"=w396:T21)  [unwired: 4 in, 2 out]
                    n183 = flat-sequence {
                      tunnel: w400 -> [w407]
                      tunnel: w399 -> [w406]
                      tunnel: [w405] -> w398
                      tunnel: [w404] -> w397
                      tunnel: w396 -> [w403]
                      tunnel: [w403] -> w394
                      tunnel: [w402] -> w393
                      frame #0 {
                        n184 = call "4G Read Mag Current.vi"("error in (no error)"=w406, "VISA session"=w407) -> ("error out"=w404:errorcluster, "response out"=w402:string, "dup VISA session"=w405:refnum<visa-resource-name>)  [unwired: 1 in]
                      }
                    }
                    n185 = Wait (ms)(milliseconds to wait=u32 500) -> ()  [unwired: 1 out]
                    n186 = call <vilib>:"Release Semaphore.vi"("semaphore"=w394) -> ()  [unwired: 5 in, 2 out]
                    n187 = Match Pattern(string=w393, regular expression="kG") -> (before substring=w391:string)  [unwired: 1 in, 3 out]
                    n188 = Fract/Exp String To Number(string=w391) -> (number=w390:dbl)  [unwired: 3 in, 1 out]
                    n189 = property on="oscillating" class="Bool (严格)"() -> ("Value"=w384:bool)  [unwired: 2 in, 2 out]
                    n190 = Multiply(x=w390, y=1000.0) -> (x*y=w388:dbl)
                    n191 = Equal?(x=w388, y=w387) -> (x = y?=w386:bool)
                    n192 = Not(x=w384) -> (.not. x?=w383:bool)
                    n193 = Or(x=w383, y=w386) -> (x .or. y?=w385:bool)
                  }
                }
                frame True {
                  n194 = call "set magnet.vi"("error in (no error)"=w411, "Magnet field(Oe)"=0.0, "semaphore"=w408, "VISA Resource Name"=w413) -> ("error out"=w410:errorcluster, "dup VISA session"=w409:refnum<visa-resource-name>)  [unwired: 5 in, 1 out]
                }
              }
              n195 = property on="oscillating" class="Bool (严格)"() -> ("Value"=w354:bool)  [unwired: 2 in, 2 out]
              n196 = Not(x=w354) -> (.not. x?=w353:bool)
              n197 = Or(x=w356, y=w353) -> (x .or. y?=w355:bool)
            }
          }
        }
        n198 = property on="oscillating" class="Bool (严格)"("Value"=w320) -> ()  [unwired: 2 in, 2 out]
      }
    }
  }
  n199 = while {
    tunnel: w1 -> [w417]
    stop <- FALSE stop-if-true
    n200 = Unbundle By Name(w417) -> ("quantum design"=w427:refnum<k24>, "340 Resource"=w426:refnum<visa-resource-name>, "Input (0:A) 340"=w425:u16, "Instrument Type"=w416:T3, "Loop (0: 1)"=w424:u16, "TCP master instance"=w423:refnum<class "Modbus Master.lvclass">, "4G supply"=w422:refnum<visa-resource-name>, "M24C Resource"=w421:refnum<visa-resource-name>, "9T信号"=w420:T21, "limit"=w419:T22, "vi路径"=w418:string)
    n201 = event shown="[23] \"树形\": 双击" {
      selector: _ -> [_ _ _ _ _ _ _ _ _ _ _ _ _ _ _ _ _ _ _ _ _ _ _ _ _]
      dyn-events: _ -> [_ _ _ _ _ _ _ _ _ _ _ _ _ _ _ _ _ _ _ _ _ _ _ _ _]
      timeout: _ -> [_ _ _ _ _ _ _ _ _ _ _ _ _ _ _ _ _ _ _ _ _ _ _ _ _]
      tunnel: w427 -> [w429 _ _ _ _ w474 _ _ _ _ w511 _ _ w582 _ _ w659 w670 _ _ _ _ _ _ _]
      tunnel: w426 -> [_ _ _ _ _ _ _ _ _ _ _ _ _ _ _ _ _ w669 _ _ _ _ _ _ _]
      tunnel: w425 -> [_ _ _ _ _ _ _ _ _ _ _ _ _ _ _ _ _ w668 _ _ _ _ _ _ _]
      tunnel: w424 -> [_ _ _ _ _ _ _ _ _ _ _ _ _ _ _ _ _ w667 _ _ _ _ _ _ _]
      tunnel: w423 -> [_ _ _ _ _ _ _ _ w501 _ _ _ _ _ _ _ _ _ _ _ _ _ _ _ w1003]
      tunnel: w422 -> [_ _ _ _ _ _ _ _ _ _ w510 _ _ _ _ _ _ _ _ _ _ _ _ _ _]
      tunnel: w421 -> [_ _ _ _ _ _ _ _ _ _ _ _ _ _ _ _ _ _ w679 _ _ _ _ _ _]
      tunnel: w420 -> [_ _ _ _ _ _ _ _ _ _ w509 _ _ _ _ _ _ _ _ _ _ _ _ _ _]
      tunnel: w419 -> [_ _ _ _ _ _ _ _ _ _ _ _ _ _ _ _ _ _ _ _ w697 _ _ w849 _]
      tunnel: w418 -> [_ _ _ _ _ _ _ _ _ _ _ _ _ _ _ _ _ _ _ _ w696 _ _ _ _]
      tunnel: w417 -> [_ w436 w444 _ _ _ w483 w490 _ w502 _ _ _ _ _ _ _ _ _ _ _ w840 _ _ _]
      tunnel: w416 -> [_ _ _ _ _ _ _ _ _ _ _ _ _ _ _ _ _ _ _ _ w695 _ _ w848 _]
      event Value Change {
        n202 = event-data() -> ()  [unwired: 1 in, 6 out]
        n203 = flat-sequence {
          tunnel: w429 -> [w431]
          frame #0 {
            n204 = Wait (ms)(milliseconds to wait=u32 100 ("等待时间（毫秒）")) -> ()  [unwired: 1 out]
            n205 = Unbundle By Name("?") -> ("Code"=w432:i32)  [unwired: 1 out]
            n206 = call "SetChamber.vi"("Code"=w432, "Instrument Ref In"=w431) -> ()  [unwired: 1 in, 3 out]
          }
          frame #1 {
            n207 = property on="chamber set" class="Bool (严格)"("Value"=FALSE ("值")) -> ()  [unwired: 2 in, 2 out]
          }
        }
      }
      event "position.In-plane": Value Change {
        n208 = event-data() -> ("CtlRef"=w435:refnum<vi>)  [unwired: 1 in, 5 out]
        n209 = property on="In plane" class="DigNum (严格)"() -> ("Value"=w437:dbl)  [unwired: 2 in, 2 out]
        n210 = flat-sequence {
          tunnel: w437 -> [w439]
          tunnel: w436 -> [w438]
          tunnel: w435 -> [w441]
          frame #0 {
            n211 = call "set in plane position.vi"("Value"=w439, "Instrument"=w438) -> ()  [unwired: 10 in]
          }
          frame #1 {
            n212 = property class="Bool (严格)"(reference=w441, "Value"=FALSE ("值")) -> ()  [unwired: 1 in, 2 out]
          }
        }
      }
      event "position.Out-plane": Value Change {
        n213 = event-data() -> ("CtlRef"=w442:refnum<vi>)  [unwired: 1 in, 5 out]
        n214 = property on="Out plane" class="DigNum (严格)"() -> ("Value"=w443:dbl)  [unwired: 2 in, 2 out]
        n215 = flat-sequence {
          tunnel: w444 -> [w446]
          tunnel: w443 -> [w445]
          tunnel: w442 -> [w448]
          frame #0 {
            n216 = call "set out plane position.vi"("Instrument"=w446, "Value"=w445) -> ()  [unwired: 10 in]
          }
          frame #1 {
            n217 = property class="Bool (严格)"(reference=w448, "Value"=FALSE ("值")) -> ()  [unwired: 1 in, 2 out]
          }
        }
      }
      event "Delete": Mouse Down {
        n218 = event-data() -> ()  [unwired: 1 in, 8 out]
        n219 = property on="列表框" class="LstBox (严格)"() -> ("Item Names"=w452:string[])  [unwired: 2 in, 2 out]
        n220 = property on="列表框" class="LstBox (严格)"() -> ("FocusRow"=w450:i32)  [unwired: 2 in, 2 out]
        n221 = Array Size(array=w452) -> (size(s)=w451:i32)
        n222 = Delete From Array(array=w452, index=w450) -> (array with subset deleted=w453:string[])  [unwired: 1 in, 1 out]
        n223 = while {
          tunnel: w451 -> [w459]
          shift-right: [w455] -> _
          shift-left: w450 -> [w456]
          tunnel: [w454] -> w449
          tunnel: w450 -> [w454]
          stop <- w458 stop-if-true
          n224 = Add(x=w456, y=1) -> (x+y=w455:i32)
          n225 = Greater Or Equal?(x=w455, y=w459) -> (x >= y?=w458:bool)
          n226 = flat-sequence {
            tunnel: w455 -> [w461]
            tunnel: [w462] -> w457
            tunnel: w456 -> [w463]
            tunnel: w457 -> [w464]
            frame #0 {
              n227 = property on="列表框" class="LstBox (严格)"("Active Row"=w461) -> ()  [unwired: 2 in, 2 out]
            }
            frame #1 {
              n228 = property on="列表框" class="LstBox (严格)"() -> ("CellFontStrike"=w462:bool)  [unwired: 2 in, 2 out]
            }
            frame #2 {
              n229 = property on="列表框" class="LstBox (严格)"("Active Row"=w463) -> ()  [unwired: 2 in, 2 out]
            }
            frame #3 {
              n230 = property on="列表框" class="LstBox (严格)"("CellFontStrike"=w464) -> ()  [unwired: 2 in, 2 out]
            }
          }
        }
        n231 = flat-sequence {
          tunnel: w453 -> [w465]
          tunnel: w450 -> [w466]
          frame #0 {
            n232 = property on="列表框" class="LstBox (严格)"("Item Names"=w465) -> ()  [unwired: 2 in, 2 out]
          }
          frame #1 {
            n233 = property on="列表框" class="LstBox (严格)"("FocusRow"=w466) -> ()  [unwired: 2 in, 2 out]
            n234 = property on="列表框" class="LstBox (严格)"("Val(Sgnl)"=w466) -> ()  [unwired: 2 in, 2 out]
          }
        }
        n235 = property on="列表框" class="LstBox (严格)"("Active Row"=w449) -> ()  [unwired: 2 in, 2 out]
      }
      event "Enable/Disable": Value Change {
        n236 = event-data() -> ()  [unwired: 1 in, 6 out]
        n237 = flat-sequence {
          frame #0 {
            n238 = property on="Enable/Disable" class="Bool (严格)"() -> ("Value"=w467:bool)  [unwired: 2 in, 2 out]
            n239 = Not(x=w467) -> (.not. x?=w468:bool)
            n240 = property on="列表框" class="LstBox (严格)"("CellFontStrike"=w468) -> ()  [unwired: 2 in, 2 out]
          }
          frame #1 {
            n241 = property on="列表框" class="LstBox (严格)"() -> ("Active Row"=w471:i32)  [unwired: 2 in, 2 out]
            n242 = Add(x=w471, y=1) -> (x+y=w469:i32)
            n243 = property on="列表框" class="LstBox (严格)"("Val(Sgnl)"=w469) -> ()  [unwired: 2 in, 2 out]
            n244 = property on="列表框" class="LstBox (严格)"("Active Row"=w469, "FocusRow"=w469) -> ()  [unwired: 2 in, 2 out]
          }
          frame #2 {
            n245 = property on="列表框" class="LstBox (严格)"() -> ("CellFontStrike"=w473:bool)  [unwired: 2 in, 2 out]
            n246 = Not(x=w473) -> (.not. x?=w472:bool)
            n247 = property on="Enable/Disable" class="Bool (严格)"("Value"=w472) -> ()  [unwired: 2 in, 2 out]
          }
        }
      }
      event Value Change {
        n248 = event-data() -> ()  [unwired: 1 in, 6 out]
        n249 = flat-sequence {
          tunnel: w474 -> [w476]
          frame #0 {
            n250 = Wait (ms)(milliseconds to wait=u32 100 ("等待时间（毫秒）")) -> ()  [unwired: 1 out]
            n251 = Unbundle By Name("?") -> ("Field"=w480:dbl, "Rate"=w479:dbl, "Mode"=w478:i32, "Approach"=w477:i32)
            n252 = call "SetField.vi"("Mode"=w478, "Approach"=w477, "Rate"=w479, "Field"=w480, "Instrument Ref In"=w476) -> ()  [unwired: 2 in, 3 out]
          }
          frame #1 {
            n253 = property on="field set" class="Bool (严格)"("Value"=FALSE ("值")) -> ()  [unwired: 2 in, 2 out]
          }
        }
      }
      event Value Change {
        n254 = event-data() -> ()  [unwired: 1 in, 6 out]
        n255 = flat-sequence {
          tunnel: w483 -> [w484]
          frame #0 {
            n256 = Unbundle By Name("?") -> ("Field(Oe)"=w487:dbl, "Rate(Oe/s）"=w486:dbl)
            n257 = call "set all (子VI).vi"("Instrument"=w484, "Rate/speed"=w486, "Target"=w487, "类型"=set_type."field") -> ()  [unwired: 7 in, 1 out]
          }
          frame #1 {
            n258 = property on="Set Field" class="Bool (严格)"("Value"=FALSE ("值")) -> ()  [unwired: 2 in, 2 out]
          }
        }
      }
      event "335 2.Set Temp": Value Change {
        n259 = event-data() -> ()  [unwired: 1 in, 6 out]
        n260 = flat-sequence {
          tunnel: w490 -> [w491]
          frame #0 {
            n261 = Unbundle By Name("335 2") -> ("Temperature"=w493:dbl, "Rate (K/min)"=w492:dbl)
            n262 = call "set all (子VI).vi"("Instrument"=w491, "Rate/speed"=w492, "Target"=w493, "类型"=set_type."temp") -> ()  [unwired: 7 in, 1 out]
          }
          frame #1 {
            n263 = property on="Set Temp" class="Bool (严格)"("Value"=FALSE ("值")) -> ()  [unwired: 2 in, 2 out]
          }
        }
      }
      event "压缩机启停": Value Change {
        n264 = event-data() -> ("NewVal"=w499:bool)  [unwired: 1 in, 5 out]
        n265 = Initialize Array(w499, 1 ("dimension size")) -> (w498:bool[])
        n266 = call-dynamic "Write Multiple Coils.vi"("coils to write"=w498, "starting address"=u16 23, "Modbus master in"=w501) -> ()  [unwired: 7 in, 2 out]
      }
      event "Position.Set Position": Value Change {
        n267 = event-data() -> ()  [unwired: 1 in, 6 out]
        n268 = flat-sequence {
          tunnel: w502 -> [w503]
          frame #0 {
            n269 = Unbundle By Name("Position") -> ("Postion"=w505:dbl, "Rate"=w504:dbl)
            n270 = call "set all (子VI).vi"("Instrument"=w503, "Rate/speed"=w504, "Target"=w505, "类型"=set_type."position") -> ()  [unwired: 7 in, 1 out]
          }
          frame #1 {
            n271 = property on="Set Position" class="Bool (严格)"("Value"=FALSE ("值")) -> ()  [unwired: 2 in, 2 out]
          }
        }
      }
      event Value Change {
        n272 = event-data() -> ()  [unwired: 1 in, 6 out]
        n273 = flat-sequence {
          tunnel: w511 -> [_]
          tunnel: w510 -> [w519]
          tunnel: w509 -> [w512]
          frame #0 {
            n274 = Wait (ms)(milliseconds to wait=u32 100 ("等待时间（毫秒）")) -> ()  [unwired: 1 out]
            n275 = Unbundle By Name("?") -> ("Field(Oe)"=w517:dbl, "Approach"=w514:enum16{"Linear", "Oscillate"}, "Rate"=w516:dbl)
            n276 = case shown="\"Linear\", 默认" w514 {
              selector: w514 -> [w521 w524]
              tunnel: [w521 w524] -> w513
              frame "Linear", Default {
                n277 = Wait (ms)(milliseconds to wait=u32 1000) -> ()  [unwired: 1 out]
                n278 = property on="oscillating" class="Bool (严格)"("Value"=FALSE ("oscillating")) -> ()  [unwired: 2 in, 2 out]
              }
              frame "Oscillate" {
              }
            }
            n279 = call "Set field (linear and oscillate).vi"("Rate(Oe/s)"=w516, "semaphore"=w512, "数值"=w517, "Approach"=w513, "VISA Resource Name"=w519) -> ("Oscillate?"=w515:bool)  [unwired: 3 in, 3 out]
            n280 = case shown="真" w515 {
              tunnel: w515 -> [_ w525]
              frame False {
              }
              frame True {
                n281 = property on="oscillating" class="Bool (严格)"("Val(Sgnl)"=w525) -> ()  [unwired: 2 in, 2 out]
              }
            }
          }
          frame #1 {
            n282 = property on="Field set" class="Bool (严格)"("Value"=FALSE ("值")) -> ()  [unwired: 2 in, 2 out]
          }
        }
      }
      event "New psr": Value Change {
        n283 = event-data() -> ()  [unwired: 1 in, 6 out]
        n284 = property on="New psr" class="Bool (严格)"("Value"=FALSE ("New psr")) -> ()  [unwired: 2 in, 2 out]
        n285 = property on="psr saved" class="Bool (严格)"() -> ("Value"=w528:bool)  [unwired: 2 in, 2 out]
        n286 = case shown="真" w528 {
          frame False {
            n287 = Two Button Dialog(message="程序尚未保存，是否放弃当前程序？" ("消息")) -> (T button?=w529:bool)  [unwired: 2 in]
            n288 = case shown="真" w529 {
              frame False {
              }
              frame True {
                n289 = property on="psr saved" class="Bool (严格)"("Value"=TRUE ("psr saved")) -> ()  [unwired: 2 in, 2 out]
                n290 = property on="New psr" class="Bool (严格)"("Val(Sgnl)"=TRUE ("New psr")) -> ()  [unwired: 2 in, 2 out]
              }
            }
          }
          frame True {
            n291 = property on="seq" class="Path"("Value"=path "") -> ()  [unwired: 2 in, 2 out]
            n292 = property on="列表框" class="LstBox (严格)"() -> ("Item Names"=w537:string[])  [unwired: 2 in, 2 out]
            n293 = Array Size(array=w537) -> (size(s)=w536:i32)
            n294 = flat-sequence {
              tunnel: w536 -> [w542]
              tunnel: [w539] -> w534
              tunnel: [w538] -> w533
              frame #0 {
                n295 = while {
                  tunnel: w542 -> [w545]
                  i -> [w548]
                  stop <- w543 stop-if-true
                  n296 = property on="列表框" class="LstBox (严格)"("CellFontStrike"=FALSE) -> ()  [unwired: 2 in, 2 out]
                  n297 = property on="列表框" class="LstBox (严格)"("Active Row"=w548) -> ()  [unwired: 2 in, 2 out]
                  n298 = Add(x=1, y=w548) -> (x+y=w546:i32)
                  n299 = Greater Or Equal?(x=w546, y=w545) -> (x >= y?=w543:bool)
                }
                n300 = property on="列表框" class="LstBox (严格)"() -> ("FocusRow"=w538:i32)  [unwired: 2 in, 2 out]
                n301 = Build Array("Initialize", "End Sequence" ("元素")) -> (w539:string[])
              }
            }
            n302 = property on="列表框" class="LstBox (严格)"("Active Row"=w533) -> ()  [unwired: 2 in, 2 out]
            n303 = property on="列表框" class="LstBox (严格)"("Item Names"=w534) -> ()  [unwired: 2 in, 2 out]
          }
        }
      }
      event "Open": Value Change {
        n304 = event-data() -> ()  [unwired: 1 in, 6 out]
        n305 = property on="Open" class="Bool (严格)"("Value"=FALSE ("open")) -> ()  [unwired: 2 in, 2 out]
        n306 = property on="psr saved" class="Bool (严格)"() -> ("Value"=w549:bool)  [unwired: 2 in, 2 out]
        n307 = case shown="真" w549 {
          frame False {
            n308 = Two Button Dialog(message="程序尚未保存，是否放弃保存当前程序？" ("消息")) -> (T button?=w551:bool)  [unwired: 2 in]
            n309 = case shown="真" w551 {
              frame False {
              }
              frame True {
                n310 = property on="psr saved" class="Bool (严格)"("Value"=TRUE ("psr saved")) -> ()  [unwired: 2 in, 2 out]
                n311 = property on="Open" class="Bool (严格)"("Val(Sgnl)"=TRUE) -> ()  [unwired: 2 in, 2 out]
              }
            }
          }
          frame True {
            n312 = Read from Text File() -> (refnum out=w558:refnum<file>, text=w561:string, error out=→"错误输出 3":errorcluster)  [unwired: 4 in, 1 out]
            n313 = while {
              shift-right: [w572] -> _
              shift-left: w561 -> [w577]
              shift-right: [w567] -> w559
              shift-left: string[] [] -> [w566]
              tunnel: [w562] -> w555
              i -> [w564]
              stop <- w573 stop-if-true
              n314 = Match Pattern(string=w577, regular expression="\n" ("正则表达式")) -> (before substring=w570:string, match substring=w571:string, after substring=w572:string)  [unwired: 1 in, 1 out]
              n315 = flat-sequence {
                tunnel: w564 -> [w578]
                tunnel: w563 -> [w579]
                frame #0 {
                  n316 = property on="列表框" class="LstBox (严格)"("Active Row"=w578) -> ()  [unwired: 2 in, 2 out]
                }
                frame #1 {
                  n317 = property on="列表框" class="LstBox (严格)"("CellFontStrike"=w579) -> ()  [unwired: 2 in, 2 out]
                }
              }
              n318 = String Length(string=w571) -> (length=w575:i32)
              n319 = Match Pattern(string=w570, regular expression=" " ("正则表达式")) -> (before substring=w568:string, after substring=w565:string)  [unwired: 1 in, 2 out]
              n320 = case shown="\"T\", 默认" w568 {
                tunnel: [TRUE FALSE] -> w563
                frame "F" {
                }
                frame "T", Default {
                }
              }
              n321 = Build Array (concatenate)(w566, w565) -> (w567:string[])
              n322 = Equal?(x=w575, y=0) -> (x = y?=w573:bool)
              n323 = property on="列表框" class="LstBox (严格)"() -> ("FocusRow"=w562:i32)  [unwired: 2 in, 2 out]
            }
            n324 = Refnum to Path(1:w558) -> (0:w557:path)
            n325 = property on="seq" class="Path"("Value"=w557) -> ()  [unwired: 2 in, 2 out]
            n326 = property on="列表框" class="LstBox (严格)"("Active Row"=w555) -> ()  [unwired: 2 in, 2 out]
            n327 = property on="列表框" class="LstBox (严格)"("Item Names"=w559) -> ()  [unwired: 2 in, 2 out]
          }
        }
      }
      event Value Change {
        n328 = event-data() -> ()  [unwired: 1 in, 6 out]
        n329 = flat-sequence {
          tunnel: w582 -> [w587]
          frame #0 {
            n330 = Wait (ms)(milliseconds to wait=u32 100 ("等待时间（毫秒）")) -> ()  [unwired: 1 out]
            n331 = Unbundle By Name("?") -> ("Position"=w586:dbl, "Mode"=w585:i32, "Speed"=w583:u16)
            n332 = call "set poisition.vi"("Mode"=w585, "Slow down code\ndefault = 0"=w583, "Position (deg)"=w586, "Instrument Ref In"=w587) -> ()  [unwired: 4 in, 2 out]
          }
          frame #1 {
            n333 = property on="position set" class="Bool (严格)"("Value"=FALSE) -> ()  [unwired: 2 in, 2 out]
          }
        }
      }
      event "Save as": Value Change {
        n334 = event-data() -> ()  [unwired: 1 in, 6 out]
        n335 = property on="Save as" class="Bool (严格)"("Value"=FALSE ("save as")) -> ()  [unwired: 2 in, 2 out]
        n336 = property on="列表框" class="LstBox (严格)"() -> ("Item Names"=w597:string[])  [unwired: 2 in, 2 out]
        n337 = Array Size(array=w597) -> (size(s)=w596:i32)
        n338 = while {
          shift-right: [w603] -> w595
          shift-left: w597 -> [w606]
          tunnel: w596 -> [w602]
          tunnel: [w601] -> w591
          i -> [w604]
          stop <- w609 stop-if-true
          n339 = Index Array(array=w606, index=w604) -> (element=w607:string)
          n340 = Add(x=w604, y=1) -> (x+y=w610:i32)
          n341 = flat-sequence {
            tunnel: w604 -> [w612]
            tunnel: [w613] -> w608
            frame #0 {
              n342 = property on="列表框" class="LstBox (严格)"("Active Row"=w612) -> ()  [unwired: 2 in, 2 out]
            }
            frame #1 {
              n343 = property on="列表框" class="LstBox (严格)"() -> ("CellFontStrike"=w614:bool)  [unwired: 2 in, 2 out]
              n344 = case shown="真" w614 {
                tunnel: ["T " "F "] -> w613
                frame False {
                }
                frame True {
                }
              }
            }
          }
          n345 = Greater Or Equal?(x=w610, y=w602) -> (x >= y?=w609:bool)
          n346 = Concatenate Strings(w608, w607) -> (w605:string)
          n347 = property on="列表框" class="LstBox (严格)"() -> ("FocusRow"=w601:i32)  [unwired: 2 in, 2 out]
          n348 = Replace Array Subset(array=w606, new element=w605, index=w604) -> (w603:string[])
        }
        n349 = Open/Create/Replace File(operation (0:open)=T26."replace or create" ("操作(0:open)")) -> (refnum out=w590:refnum<file>, error out=w594:errorcluster)  [unwired: 5 in, 1 out]
        n350 = property on="列表框" class="LstBox (严格)"("Active Row"=w591) -> ()  [unwired: 2 in, 2 out]
        n351 = Write to Text File(file (use dialog)=w590, text=w595, error in=w594) -> (refnum out=w598:refnum<file>, error out=w593:errorcluster)  [unwired: 1 in, 1 out]
        n352 = Close File(refnum=w598, error in=w593) -> (error out=→"错误输出":errorcluster)  [unwired: 1 out]
      }
      event "Save": Value Change {
        n353 = event-data() -> ()  [unwired: 1 in, 6 out]
        n354 = property on="Save" class="Bool (严格)"("Value"=FALSE ("save")) -> ()  [unwired: 2 in, 2 out]
        n355 = property on="psr saved" class="Bool (严格)"("Value"=TRUE ("psr saved")) -> ()  [unwired: 2 in, 2 out]
        n356 = property on="列表框" class="LstBox (严格)"() -> ("Item Names"=w620:string[])  [unwired: 2 in, 2 out]
        n357 = Array Size(array=w620) -> (size(s)=w621:i32)
        n358 = while {
          shift-right: [w629] -> w622
          shift-left: w620 -> [w632]
          tunnel: w621 -> [w628]
          tunnel: [w627] -> w619
          i -> [w630]
          stop <- w635 stop-if-true
          n359 = Index Array(array=w632, index=w630) -> (element=w633:string)
          n360 = Add(x=w630, y=1) -> (x+y=w636:i32)
          n361 = flat-sequence {
            tunnel: w630 -> [w638]
            tunnel: [w639] -> w634
            frame #0 {
              n362 = property on="列表框" class="LstBox (严格)"("Active Row"=w638) -> ()  [unwired: 2 in, 2 out]
            }
            frame #1 {
              n363 = property on="列表框" class="LstBox (严格)"() -> ("CellFontStrike"=w640:bool)  [unwired: 2 in, 2 out]
              n364 = case shown="真" w640 {
                tunnel: ["T " "F "] -> w639
                frame False {
                }
                frame True {
                }
              }
            }
          }
          n365 = Greater Or Equal?(x=w636, y=w628) -> (x >= y?=w635:bool)
          n366 = Concatenate Strings(w634, w633) -> (w631:string)
          n367 = property on="列表框" class="LstBox (严格)"() -> ("FocusRow"=w627:i32)  [unwired: 2 in, 2 out]
          n368 = Replace Array Subset(array=w632, new element=w631, index=w630) -> (w629:string[])
        }
        n369 = property on="seq" class="Path"() -> ("Value"=w617:path)  [unwired: 2 in, 2 out]
        n370 = Path To String(path=w617) -> (string=w624:string)
        n371 = String Length(string=w624) -> (length=w623:i32)
        n372 = property on="列表框" class="LstBox (严格)"("Active Row"=w619) -> ()  [unwired: 2 in, 2 out]
        n373 = case shown="1, 默认" w623 {
          tunnel: w622 -> [w648 w658]
          tunnel: T26."replace or create" ("操作(0:open)") -> [w647 w654]
          tunnel: w617 -> [_ w651]
          frame 0 {
            n374 = Open/Create/Replace File(operation (0:open)=w647) -> (refnum out=w646:refnum<file>, error out=w645:errorcluster)  [unwired: 5 in, 1 out]
            n375 = Write to Text File(file (use dialog)=w646, text=w648, error in=w645) -> (refnum out=w650:refnum<file>, error out=w644:errorcluster)  [unwired: 1 in, 1 out]
            n376 = Close File(refnum=w650, error in=w644) -> (path=w649:path, error out=→"错误输出 4":errorcluster)
            n377 = property on="seq" class="Path"("Value"=w649) -> ()  [unwired: 2 in, 2 out]
          }
          frame 1, Default {
            n378 = Open/Create/Replace File(file path (use dialog)=w651, operation (0:open)=w654) -> (refnum out=w652:refnum<file>, error out=w653:errorcluster)  [unwired: 4 in, 1 out]
            n379 = Write to Text File(file (use dialog)=w652, text=w658, error in=w653) -> (refnum out=w657:refnum<file>, error out=w656:errorcluster)  [unwired: 1 in, 1 out]
            n380 = Close File(refnum=w657, error in=w656) -> (error out=→"错误输出 2":errorcluster)  [unwired: 1 out]
          }
        }
      }
      event Value Change {
        n381 = event-data() -> ()  [unwired: 1 in, 6 out]
        n382 = flat-sequence {
          tunnel: w659 -> [w661]
          frame #0 {
            n383 = Wait (ms)(milliseconds to wait=u32 100 ("等待时间（毫秒）")) -> ()  [unwired: 1 out]
            n384 = Unbundle By Name("?") -> ("Temperature"=w664:dbl, "Rate"=w663:dbl, "Mode"=w662:i32)
            n385 = call "SetTemperature.vi"("Approach"=w662, "Rate"=w663, "Temperature"=w664, "Instrument Ref In"=w661) -> ()  [unwired: 3 in, 3 out]
          }
          frame #1 {
            n386 = property on="temp set" class="Bool (严格)"("Value"=FALSE ("值")) -> ()  [unwired: 2 in, 2 out]
          }
        }
      }
      event Value Change {
        n387 = event-data() -> ()  [unwired: 1 in, 6 out]
        n388 = flat-sequence {
          tunnel: w670 -> [_]
          tunnel: w669 -> [w676]
          tunnel: w668 -> [w672]
          tunnel: w667 -> [w671]
          frame #0 {
            n389 = Wait (ms)(milliseconds to wait=u32 100 ("等待时间（毫秒）")) -> ()  [unwired: 1 out]
            n390 = Unbundle By Name("?") -> ("Temperature"=w674:dbl, "Rate"=w673:dbl)
            n391 = call "325 set Temp(SubVI).vi"("Output (1:1)"=w672, "Input (0:A)"=w671, "Rate"=w673, "Temperature"=w674, "VISA Refnum in"=w676) -> ()  [unwired: 5 in, 2 out]
          }
          frame #1 {
            n392 = property on="temp set" class="Bool (严格)"("Value"=FALSE ("值")) -> ()  [unwired: 2 in, 2 out]
          }
        }
      }
      event Value Change {
        n393 = event-data() -> ()  [unwired: 1 in, 6 out]
        n394 = flat-sequence {
          tunnel: w679 -> [w684]
          frame #0 {
            n395 = Wait (ms)(milliseconds to wait=u32 100 ("等待时间（毫秒）")) -> ()  [unwired: 1 out]
            n396 = Unbundle By Name("?") -> ("Temperature"=w682:dbl, "Rate"=w683:dbl, "Ctrl On"=w680:bool)
            n397 = call "set 24C temp(SubVI).vi"("Control"=w680, "Temperature"=w682, "Rate"=w683, "VISA引用句柄输入"=w684) -> ()  [unwired: 7 in, 1 out]
          }
          frame #1 {
            n398 = property on="Temp set" class="Bool (严格)"("Value"=FALSE ("值")) -> ()  [unwired: 2 in, 2 out]
          }
        }
      }
      event "列表框": Mouse Down {
        n399 = event-data() -> ()  [unwired: 1 in, 8 out]
        n400 = flat-sequence {
          frame #0 {
            n401 = property on="列表框" class="LstBox (严格)"() -> ("FocusRow"=w687:i32)  [unwired: 2 in, 2 out]
            n402 = property on="列表框" class="LstBox (严格)"("Active Row"=w687) -> ()  [unwired: 2 in, 2 out]
          }
          frame #1 {
            n403 = property on="列表框" class="LstBox (严格)"() -> ("CellFontStrike"=w689:bool)  [unwired: 2 in, 2 out]
            n404 = Not(x=w689) -> (.not. x?=w688:bool)
            n405 = property on="Enable/Disable" class="Bool (严格)"("Value"=w688) -> ()  [unwired: 2 in, 2 out]
          }
        }
      }
      event "列表框": Double Click {
        n406 = event-data() -> ()  [unwired: 1 in, 9 out]
        n407 = property on="列表框" class="LstBox (严格)"() -> ("Item Names"=w700:string[])  [unwired: 2 in, 2 out]
        n408 = property on="列表框" class="LstBox (严格)"() -> ("FocusRow"=w701:i32)  [unwired: 2 in, 2 out]
        n409 = Index Array(array=w700, index=w701) -> (element=w694:string)
        n410 = call "how_many_indentation.vi"("input"=w694) -> ("indentation"=w690:string, "remain"=w692:string)  [unwired: 9 in]
        n411 = call "string front part.vi"("字符串"=w692, "偏移量(0)"=7) -> ("result string"=w698:string)  [unwired: 9 in]
        n412 = case shown="\"Initial\"" w698 {
          tunnel: [w711 w714 w724 w765 w767 w776 w778 w780 w784 w788 w791 w793 w805 w808 w810 w813 w816 w818 w821 w826 w830 w833 "" ("连接的字符串")] -> w691
          tunnel: [w710 w713 w725 w764 w766 w775 w777 w779 w783 w787 w790 w792 w804 w807 w811 w812 w815 w817 w820 w825 w829 w832 FALSE ("布尔 3")] -> w702
          tunnel: w692 -> [w712 w715 w722 w763 w768 _ _ w781 w782 w786 w789 w794 w803 w806 w809 _ w814 w819 w822 w824 w828 w831 _]
          tunnel: w697 -> [_ _ _ _ _ _ _ _ _ w785 _ _ w802 _ _ _ _ _ _ w823 w827 _ _]
          tunnel: w696 -> [_ _ w719 _ _ _ _ _ _ _ _ _ _ _ _ _ _ _ _ _ _ _ _]
          tunnel: w695 -> [_ _ _ _ w769 _ _ _ _ _ _ w795 _ _ _ _ _ _ _ _ _ _ _]
          frame "Delta d" {
            n413 = call "add delta delay(SubVI).vi"("字符串"=w712) -> ("ok or cancel"=w710:bool, "连接的字符串"=w711:string)  [unwired: 9 in]
          }
          frame "Delta r" {
            n414 = call "add delta range(SubVI).vi"("字符串"=w715) -> ("ok or cancel"=w713:bool, "连接的字符串"=w714:string)  [unwired: 9 in]
          }
          frame "Initial" {
            n415 = Match Pattern(string=w722, regular expression="Initialize " ("正则表达式")) -> (after substring=w717:string)  [unwired: 1 in, 3 out]
            n416 = Match Pattern(string=w717, regular expression=" model " ("正则表达式")) -> (before substring=w716:string, after substring=w718:string)  [unwired: 1 in, 2 out]
            n417 = Concatenate Strings(w719, w718) -> (w720:string)
            n418 = case shown="\"4200\"" w716 {
              selector: w716 -> [_ _ _ w741 w742 w746 w750 w756 _]
              tunnel: w720 -> [w729 w732 w737 w740 w745 w749 w754 w755 w762]
              tunnel: [w728 w730 w736 w738 w744 w747 w753 w759 w761] -> w725
              tunnel: [w727 w731 w735 w739 w743 w748 w752 w758 w760] -> w724
              frame "Delta" {
                n419 = call "add delta initalize(SubVI).vi"("字符串"=w729, "model"="Delta") -> ("连接的字符串"=w727:string, "ok or cancel"=w728:bool)  [unwired: 8 in]
              }
              frame "4200" {
                n420 = call "add 4200 initalize(SubVI).vi"("字符串"=w732, "model"="4200") -> ("连接的字符串"=w731:string, "ok or cancel"=w730:bool)  [unwired: 8 in]
              }
              frame "Delta-tunnelling", Default {
                n421 = call "add delta initalize(SubVI).vi"("字符串"=w737, "model"="Delta-tunnelling") -> ("连接的字符串"=w735:string, "ok or cancel"=w736:bool)  [unwired: 8 in]
              }
              frame "keithley6221-2182-DC" {
                n422 = call "add 6221-2182-DC initalize(SubVI).vi"("字符串"=w740, "model"=w741) -> ("连接的字符串"=w739:string, "ok or cancel"=w738:bool)  [unwired: 8 in]
              }
              frame "Gating" {
                n423 = call "add gating initalize(SubVI).vi"("字符串"=w745, "model"=w742) -> ("连接的字符串"=w743:string, "ok or cancel"=w744:bool)  [unwired: 8 in]
              }
              frame "Dual-gating" {
                n424 = call "add dual gating initalize(SubVI).vi"("字符串"=w749, "model"=w746) -> ("连接的字符串"=w748:string, "ok or cancel"=w747:bool)  [unwired: 8 in]
              }
              frame "keithley6221-SR830" {
                n425 = call "add SR830 initalize(SubVI).vi"("字符串"=w754, "model"=w750, "6221"=TRUE) -> ("连接的字符串"=w752:string, "ok or cancel"=w753:bool)  [unwired: 5 in]
              }
              frame "SR830" {
                n426 = call "add SR830 initalize(SubVI).vi"("字符串"=w755, "model"=w756, "6221"=FALSE) -> ("连接的字符串"=w758:string, "ok or cancel"=w759:bool)  [unwired: 5 in]
              }
              frame "PZT" {
                n427 = call "add PZT initalize(SubVI).vi"("字符串"=w762) -> ("连接的字符串"=w760:string, "ok or cancel"=w761:bool)  [unwired: 9 in]
              }
            }
          }
          frame "LogData" {
            n428 = call "add logppms(SubVI).vi"("字符串"=w763) -> ("ok or cancel"=w764:bool, "连接的字符串"=w765:string)  [unwired: 9 in]
          }
          frame "Move Sa" {
            n429 = case shown="\"PPMS\", 默认" w769 {
              tunnel: [w771 w774] -> w767
              tunnel: [w770 w773] -> w766
              tunnel: w768 -> [_ w772]
              frame "PPMS", Default {
                n430 = call "add set position(SubVI).vi"() -> ("布尔 3"=w770:bool, "连接的字符串"=w771:string)  [unwired: 10 in]
              }
              frame "9T mag" {
                n431 = call "add set cmag position(SubVI).vi"("字符串"=w772) -> ("布尔 3"=w773:bool, "连接的字符串"=w774:string)  [unwired: 9 in]
              }
            }
          }
          frame "Measure" {
            n432 = call "add measure(SubVI).vi"() -> ("ok or cancel"=w775:bool, "连接的字符串"=w776:string)  [unwired: 10 in]
          }
          frame "Open SR" {
            n433 = call "add open sr830(SubVI).vi"() -> ("ok or cancel"=w777:bool, "open"=w778:string)  [unwired: 10 in]
          }
          frame "PZT Tem" {
            n434 = call "add scan PZT at temp.vi"("字符串"=w781) -> ("ok or cancel"=w779:bool, "连接的字符串"=w780:string)  [unwired: 9 in]
          }
          frame "Scan Cu" {
            n435 = call "add scan current(SubVI).vi"("字符串"=w782) -> ("ok or cancel"=w783:bool, "连接的字符串"=w784:string)  [unwired: 9 in]
          }
          frame "Scan Fi" {
            n436 = call "add scan field(SubVI).vi"("limit"=w785, "字符串"=w786) -> ("布尔 3"=w787:bool, "连接的字符串"=w788:string)  [unwired: 8 in]
          }
          frame "Scan PZ" {
            n437 = call "add scan PZT V(SubVI).vi"("字符串"=w789) -> ("ok or cancel"=w790:bool, "连接的字符串"=w791:string)  [unwired: 9 in]
          }
          frame "Scan Po" {
            n438 = case shown="\"VersaLab\", 默认" w795 {
              tunnel: [w798 w801] -> w793
              tunnel: [w797 w800] -> w792
              tunnel: w794 -> [w796 w799]
              frame "9T mag" {
                n439 = call "add cmag scan position(SubVI).vi"("字符串"=w796) -> ("布尔 3"=w797:bool, "连接的字符串"=w798:string)  [unwired: 9 in]
              }
              frame "VersaLab", Default {
                n440 = call "add scan position(SubVI).vi"("字符串"=w799) -> ("布尔 3"=w800:bool, "连接的字符串"=w801:string)  [unwired: 9 in]
              }
            }
          }
          frame "Scan Te" {
            n441 = call "add scan temp(SubVI).vi"("limit"=w802, "字符串"=w803) -> ("布尔 3"=w804:bool, "连接的字符串"=w805:string)  [unwired: 8 in]
          }
          frame "Scan Ti" {
            n442 = call "add scan time(SubVI).vi"("字符串"=w806) -> ("ok or cancel"=w807:bool, "连接的字符串"=w808:string)  [unwired: 9 in]
          }
          frame "Select " {
            n443 = call "add select channel(SubVI).vi"("字符串"=w809) -> ("连接的字符串"=w810:string, "ok or cancel"=w811:bool)  [unwired: 9 in]
          }
          frame "Set Cur" {
            n444 = call "add set current(SubVI).vi"() -> ("ok or cancel"=w812:bool, "连接的字符串"=w813:string)  [unwired: 10 in]
          }
          frame "Set Dat" {
            n445 = call "add datafile(SubVI).vi"("字符串"=w814) -> ("ok or cancel"=w815:bool, "连接的字符串"=w816:string)  [unwired: 9 in]
          }
          frame "Set Gat" {
            n446 = call "add set gating(SubVI).vi"("字符串"=w819) -> ("ok or cancel"=w817:bool, "连接的字符串"=w818:string)  [unwired: 9 in]
          }
          frame "Scan Ga" {
            n447 = call "add scan gating(SubVI).vi"("字符串"=w822) -> ("布尔 3"=w820:bool, "连接的字符串"=w821:string)  [unwired: 9 in]
          }
          frame "Set Mag" {
            n448 = call "add set field(SubVI).vi"("limit"=w823, "字符串"=w824) -> ("布尔 3"=w825:bool, "连接的字符串"=w826:string)  [unwired: 8 in]
          }
          frame "Set Tem" {
            n449 = call "add set temp(SubVI).vi"("limit"=w827, "字符串"=w828) -> ("布尔 3"=w829:bool, "连接的字符串"=w830:string)  [unwired: 8 in]
          }
          frame "Wait Fo" {
            n450 = call "add wait(SubVI).vi"("字符串"=w831) -> ("ok or cancel"=w832:bool, "连接的字符串"=w833:string)  [unwired: 9 in]
          }
          frame "假", Default {
          }
        }
        n451 = Concatenate Strings(w690, w691) -> (w693:string)
        n452 = case shown="真" w702 {
          tunnel: w693 -> [_ w704]
          frame False {
          }
          frame True {
            n453 = flat-sequence {
              tunnel: w704 -> [w708]
              tunnel: [w706] -> w703
              tunnel: w703 -> [w709]
              frame #0 {
                n454 = property on="列表框" class="LstBox (严格)"() -> ("Item Names"=w705:string[])  [unwired: 2 in, 2 out]
                n455 = property on="列表框" class="LstBox (严格)"() -> ("FocusRow"=w706:i32)  [unwired: 2 in, 2 out]
                n456 = Array Size(array=w705) -> ()  [unwired: 1 out]
                n457 = Replace Array Subset(array=w705, new element=w708, index=w706) -> (w707:string[])
                n458 = property on="列表框" class="LstBox (严格)"("Item Names"=w707) -> ()  [unwired: 2 in, 2 out]
              }
              frame #1 {
                n459 = property on="列表框" class="LstBox (严格)"("FocusRow"=w709) -> ()  [unwired: 2 in, 2 out]
                n460 = property on="列表框" class="LstBox (严格)"("Val(Sgnl)"=w709) -> ()  [unwired: 2 in, 2 out]
              }
            }
          }
        }
      }
      event "行数": Value Change {
        n461 = event-data() -> ("NewVal"=w837:i32)  [unwired: 1 in, 5 out]
        n462 = Unbundle By Name(w840) -> ("列表框"=w839:refnum<vi>)
        n463 = property class="LstBox (严格)"(reference=w839) -> ("Item Names"=w838:string[])  [unwired: 1 in, 2 out]
        n464 = Index Array(array=w838, index=w837) -> (element=→"?":string)
      }
      event "列表框": Value Change {
        n465 = event-data() -> ()  [unwired: 1 in, 6 out]
        n466 = local write "编辑列表框"(TRUE) -> ()
        n467 = property on="列表框" class="LstBox (严格)"("SelColor"=u32 255 ("选择颜色 3")) -> ()  [unwired: 2 in, 2 out]
        n468 = property on="psr saved" class="Bool (严格)"("Value"=FALSE ("psr saved")) -> ()  [unwired: 2 in, 2 out]
      }
      event "树形": Double Click {
        n469 = event-data() -> ()  [unwired: 1 in, 8 out]
        n470 = case shown="\"Auto Range\"" "树形" {
          tunnel: [FALSE ("布尔 3") w910 w912 w915 w918 w922 w924 w925 w930 w931 w937 w939 w943 w944 w946 w950 w952 w956 w957 TRUE ("ok or cancel") TRUE ("ok or cancel") TRUE ("ok or cancel") w965 w967 w969 w971 w973 w976 w983 w989 w991 w993 w995 w997 w1000 w1001] -> w851
          tunnel: ["" ("连接的字符串") w909 w911 w914 w917 w921 w923 w926 w929 w932 w936 w940 w942 w945 w947 w949 w953 w955 w958 "End Sequence" "Auto Range" "Initialize" ("连接的字符串") w966 w968 w970 w972 w974 w977 w984 w990 w992 w994 w996 w998 w999 w1002] -> w850
          tunnel: w849 -> [_ _ _ _ _ _ _ _ _ _ _ w938 w941 _ _ w948 w951 _ _ _ _ _ _ _ _ _ _ _ _ _ _ _ _ _ _ _]
          tunnel: w848 -> [_ _ _ _ _ _ _ _ _ _ _ _ _ _ _ _ _ _ _ _ _ _ _ _ _ _ _ w975 w982 _ _ _ _ _ _ _]
          frame "假", Default {
          }
          frame "normal delta" {
            n471 = call "add delta initalize(SubVI).vi"("model"="Delta") -> ("连接的字符串"=w909:string, "ok or cancel"=w910:bool)  [unwired: 9 in]
          }
          frame "Delta tunnelling" {
            n472 = call "add delta initalize(SubVI).vi"("model"="Delta-tunnelling") -> ("连接的字符串"=w911:string, "ok or cancel"=w912:bool)  [unwired: 9 in]
          }
          frame "keithley2400-gating" {
            n473 = call "add gating initalize(SubVI).vi"("model"="Gating") -> ("连接的字符串"=w914:string, "ok or cancel"=w915:bool)  [unwired: 9 in]
          }
          frame "keithley6221-2182-DC" {
            n474 = call "add 6221-2182-DC initalize(SubVI).vi"("model"="keithley6221-2182-DC") -> ("连接的字符串"=w917:string, "ok or cancel"=w918:bool)  [unwired: 9 in]
          }
          frame "2614b-dual gating" {
            n475 = call "add dual gating initalize(SubVI).vi"("model"="Dual-gating") -> ("连接的字符串"=w921:string, "ok or cancel"=w922:bool)  [unwired: 9 in]
          }
          frame "PZT" {
            n476 = call "add PZT initalize(SubVI).vi"() -> ("连接的字符串"=w923:string, "ok or cancel"=w924:bool)  [unwired: 10 in]
          }
          frame "PZT Temp" {
            n477 = call "add scan PZT at temp.vi"() -> ("ok or cancel"=w925:bool, "连接的字符串"=w926:string)  [unwired: 10 in]
          }
          frame "keithley6221-SR830" {
            n478 = call "add SR830 initalize(SubVI).vi"("model"="keithley6221-SR830", "6221"=TRUE) -> ("连接的字符串"=w929:string, "ok or cancel"=w930:bool)  [unwired: 6 in]
          }
          frame "SR830" {
            n479 = call "add SR830 initalize(SubVI).vi"("model"="SR830", "6221"=FALSE) -> ("连接的字符串"=w932:string, "ok or cancel"=w931:bool)  [unwired: 6 in]
          }
          frame "tunnelling" {
            n480 = call "add delta initalize(SubVI).vi"("model"="Delta-tunnelling") -> ("连接的字符串"=w936:string, "ok or cancel"=w937:bool)  [unwired: 9 in]
          }
          frame "Set Field" {
            n481 = call "add set field(SubVI).vi"("limit"=w938) -> ("布尔 3"=w939:bool, "连接的字符串"=w940:string)  [unwired: 9 in]
          }
          frame "Set Temp" {
            n482 = call "add set temp(SubVI).vi"("limit"=w941) -> ("布尔 3"=w943:bool, "连接的字符串"=w942:string)  [unwired: 9 in]
          }
          frame "Delta delay" {
            n483 = call "add delta delay(SubVI).vi"() -> ("ok or cancel"=w944:bool, "连接的字符串"=w945:string)  [unwired: 10 in]
          }
          frame "Delta range" {
            n484 = call "add delta range(SubVI).vi"() -> ("ok or cancel"=w946:bool, "连接的字符串"=w947:string)  [unwired: 10 in]
          }
          frame "Scan Field" {
            n485 = call "add scan field(SubVI).vi"("limit"=w948) -> ("布尔 3"=w950:bool, "连接的字符串"=w949:string)  [unwired: 9 in]
          }
          frame "Scan Temp" {
            n486 = call "add scan temp(SubVI).vi"("limit"=w951) -> ("布尔 3"=w952:bool, "连接的字符串"=w953:string)  [unwired: 9 in]
          }
          frame "keithley4200" {
            n487 = call "add 4200 initalize(SubVI).vi"("model"="4200") -> ("连接的字符串"=w955:string, "ok or cancel"=w956:bool)  [unwired: 9 in]
          }
          frame "Wait" {
            n488 = call "add wait(SubVI).vi"() -> ("ok or cancel"=w957:bool, "连接的字符串"=w958:string)  [unwired: 10 in]
          }
          frame "end" {
          }
          frame "Auto Range" {
          }
          frame "initialize" {
          }
          frame "datafile" {
            n489 = call "add datafile(SubVI).vi"() -> ("ok or cancel"=w965:bool, "连接的字符串"=w966:string)  [unwired: 10 in]
          }
          frame "remark" {
            n490 = call "add remark(SubVI).vi"() -> ("ok or cancel"=w967:bool, "连接的字符串"=w968:string)  [unwired: 10 in]
          }
          frame "Scan Time" {
            n491 = call "add scan time(SubVI).vi"() -> ("ok or cancel"=w969:bool, "连接的字符串"=w970:string)  [unwired: 10 in]
          }
          frame "Scan PZT V" {
            n492 = call "add scan PZT V(SubVI).vi"() -> ("ok or cancel"=w971:bool, "连接的字符串"=w972:string)  [unwired: 10 in]
          }
          frame "logppms" {
            n493 = call "add logppms(SubVI).vi"() -> ("ok or cancel"=w973:bool, "连接的字符串"=w974:string)  [unwired: 10 in]
          }
          frame "Scan Position" {
            n494 = case shown="\"VersaLab\", 默认" w975 {
              tunnel: [w979 w981] -> w977
              tunnel: [w978 w980] -> w976
              frame "9T mag" {
                n495 = call "add cmag scan position(SubVI).vi"() -> ("布尔 3"=w978:bool, "连接的字符串"=w979:string)  [unwired: 10 in]
              }
              frame "VersaLab", Default {
                n496 = call "add scan position(SubVI).vi"() -> ("布尔 3"=w980:bool, "连接的字符串"=w981:string)  [unwired: 10 in]
              }
            }
          }
          frame "Set Position" {
            n497 = case shown="\"PPMS\", \"lengtou2\", 默认" w982 {
              tunnel: [w986 w988] -> w984
              tunnel: [w985 w987] -> w983
              frame "PPMS", "lengtou2", Default {
                n498 = call "add set position(SubVI).vi"() -> ("布尔 3"=w985:bool, "连接的字符串"=w986:string)  [unwired: 10 in]
              }
              frame "9T mag" {
                n499 = call "add set cmag position(SubVI).vi"() -> ("布尔 3"=w987:bool, "连接的字符串"=w988:string)  [unwired: 10 in]
              }
            }
          }
          frame "Set Current" {
            n500 = call "add set current(SubVI).vi"() -> ("ok or cancel"=w989:bool, "连接的字符串"=w990:string)  [unwired: 10 in]
          }
          frame "Open" {
            n501 = call "add open sr830(SubVI).vi"() -> ("ok or cancel"=w991:bool, "open"=w992:string)  [unwired: 10 in]
          }
          frame "Scan Current" {
            n502 = call "add scan current(SubVI).vi"() -> ("ok or cancel"=w993:bool, "连接的字符串"=w994:string)  [unwired: 10 in]
          }
          frame "Set Gating" {
            n503 = call "add set gating(SubVI).vi"() -> ("ok or cancel"=w995:bool, "连接的字符串"=w996:string)  [unwired: 10 in]
          }
          frame "Scan Gating" {
            n504 = call "add scan gating(SubVI).vi"() -> ("布尔 3"=w997:bool, "连接的字符串"=w998:string)  [unwired: 10 in]
          }
          frame "Select Channel" {
            n505 = call "add select channel(SubVI).vi"() -> ("连接的字符串"=w999:string, "ok or cancel"=w1000:bool)  [unwired: 10 in]
          }
          frame "measure" {
            n506 = call "add measure(SubVI).vi"() -> ("ok or cancel"=w1001:bool, "连接的字符串"=w1002:string)  [unwired: 10 in]
          }
        }
        n507 = call "string front part.vi"("字符串"="树形", "偏移量(0)"=4) -> ("result string"=w845:string)  [unwired: 9 in]
        n508 = case shown="\"Scan\"" w845 {
          tunnel: [FALSE TRUE] -> w844
          frame "假", Default {
          }
          frame "Scan" {
          }
        }
        n509 = case shown="真" w851 {
          tunnel: w850 -> [_ w865]
          tunnel: w844 -> [_ w862]
          frame False {
          }
          frame True {
            n510 = property on="列表框" class="LstBox (严格)"() -> ("Item Names"=w867:string[])  [unwired: 2 in, 2 out]
            n511 = property on="列表框" class="LstBox (严格)"() -> ("FocusRow"=w860:i32)  [unwired: 2 in, 2 out]
            n512 = Index Array(array=w867, index=w860) -> (element=w866:string)
            n513 = call "how_many_indentation.vi"("input"=w866) -> ("indentation"=w861:string)  [unwired: 9 in, 1 out]
            n514 = Concatenate Strings(w861, w865) -> (w864:string)
            n515 = Insert Into Array(array=w867, index=w860, new element=w864) -> (w863:string[])
            n516 = case shown="假" w862 {
              tunnel: w863 -> [w869 w879]
              tunnel: [w869 w878] -> w859
              tunnel: w860 -> [_ w877]
              tunnel: [1 ("y") 2 ("y")] -> w857
              tunnel: w861 -> [_ w874]
              tunnel: [w868 w871] -> w858
              frame False {
                n517 = Array Size(array=w869) -> (size(s)=w868:i32)
              }
              frame True {
                n518 = Increment(x=w877) -> (x+1=w876:i32)
                n519 = Concatenate Strings(w874, "End Scan" ("新元素/子数组")) -> (w872:string)
                n520 = Insert Into Array(array=w879, index=w876, new element=w872) -> (w878:string[])
                n521 = Array Size(array=w878) -> (size(s)=w871:i32)
              }
            }
            n522 = Add(x=w860, y=w857) -> (x+y=w856:i32)
            n523 = flat-sequence {
              tunnel: w859 -> [w880]
              tunnel: w856 -> [w881]
              tunnel: [w881] -> w855
              tunnel: w858 -> [w886]
              tunnel: w857 -> [w884]
              tunnel: w855 -> [w883]
              tunnel: [w882] -> w854
              tunnel: w854 -> [w899]
              frame #0 {
                n524 = property on="列表框" class="LstBox (严格)"("Item Names"=w880) -> ()  [unwired: 2 in, 2 out]
              }
              frame #1 {
                n525 = property on="列表框" class="LstBox (严格)"("FocusRow"=w881) -> ()  [unwired: 2 in, 2 out]
                n526 = property on="列表框" class="LstBox (严格)"("Val(Sgnl)"=w881) -> ()  [unwired: 2 in, 2 out]
              }
              frame #2 {
                n527 = Decrement(x=w886) -> (x-1=w885:i32)
                n528 = while {
                  shift-right: [w890] -> w882
                  shift-left: w885 -> [w889]
                  tunnel: w884 -> [w891]
                  tunnel: w883 -> [w888]
                  stop <- w887 stop-if-true
                  n529 = Subtract(x=w889, y=w891) -> (x-y=w892:i32)
                  n530 = flat-sequence {
                    tunnel: w892 -> [w894]
                    tunnel: [w895] -> w893
                    tunnel: w889 -> [w896]
                    tunnel: w893 -> [w897]
                    frame #0 {
                      n531 = property on="列表框" class="LstBox (严格)"("Active Row"=w894) -> ()  [unwired: 2 in, 2 out]
                    }
                    frame #1 {
                      n532 = property on="列表框" class="LstBox (严格)"() -> ("CellFontStrike"=w895:bool)  [unwired: 2 in, 2 out]
                    }
                    frame #2 {
                      n533 = property on="列表框" class="LstBox (严格)"("Active Row"=w896) -> ()  [unwired: 2 in, 2 out]
                    }
                    frame #3 {
                      n534 = property on="列表框" class="LstBox (严格)"("CellFontStrike"=w897) -> ()  [unwired: 2 in, 2 out]
                    }
                  }
                  n535 = Decrement(x=w889) -> (x-1=w890:i32)
                  n536 = Equal?(x=w889, y=w888) -> (x = y?=w887:bool)
                }
              }
              frame #3 {
                n537 = flat-sequence {
                  tunnel: w899 -> [w901]
                  tunnel: w900 -> [w903]
                  tunnel: w898 -> [w905]
                  frame #0 {
                    n538 = property on="列表框" class="LstBox (严格)"("Active Row"=w901) -> ()  [unwired: 2 in, 2 out]
                  }
                  frame #1 {
                    n539 = property on="列表框" class="LstBox (严格)"("CellFontStrike"=FALSE ("活动行:单元格字体:删除线")) -> ()  [unwired: 2 in, 2 out]
                  }
                  frame #2 {
                    n540 = property on="列表框" class="LstBox (严格)"("Active Row"=w903) -> ()  [unwired: 2 in, 2 out]
                  }
                  frame #3 {
                    n541 = property on="列表框" class="LstBox (严格)"("CellFontStrike"=FALSE ("活动行:单元格字体:删除线")) -> ()  [unwired: 2 in, 2 out]
                  }
                  frame #4 {
                    n542 = property on="列表框" class="LstBox (严格)"("Active Row"=w905) -> ()  [unwired: 2 in, 2 out]
                  }
                }
                n543 = Increment(x=w899) -> (x+1=w898:i32)
                n544 = Decrement(x=w899) -> (x-1=w900:i32)
              }
            }
          }
        }
      }
      event "压缩机开启": Value Change {
        n545 = event-data() -> ("NewVal"=w1004:bool)  [unwired: 1 in, 5 out]
        n546 = flat-sequence {
          tunnel: w1004 -> [w1005]
          tunnel: w1003 -> [w1007]
          frame #0 {
            n547 = case shown="假" w1005 {
              selector: w1005 -> [w1010 w1018]
              tunnel: w1007 -> [w1009 w1016]
              frame False {
                n548 = Build Array(w1010) -> (w1012:bool[])
                n549 = call-dynamic "Write Multiple Coils.vi"("coils to write"=w1012, "starting address"=u16 23, "Modbus master in"=w1009) -> ("Modbus master out"=w1011:refnum<class "Modbus Master.lvclass">)  [unwired: 7 in, 1 out]
                n550 = call-dynamic "Write Multiple Coils.vi"("coils to write"=w1012, "starting address"=u16 22, "Modbus master in"=w1011) -> ()  [unwired: 7 in, 2 out]
              }
              frame True {
                n551 = Build Array(w1018) -> (w1017:bool[])
                n552 = call-dynamic "Write Multiple Coils.vi"("coils to write"=w1017, "starting address"=u16 22, "Modbus master in"=w1016) -> ("Modbus master out"=w1015:refnum<class "Modbus Master.lvclass">)  [unwired: 7 in, 1 out]
                n553 = call-dynamic "Write Multiple Coils.vi"("coils to write"=w1017, "starting address"=u16 23, "Modbus master in"=w1015) -> ()  [unwired: 7 in, 2 out]
              }
            }
            n554 = Wait (ms)(milliseconds to wait=u32 100 ("等待时间（毫秒）")) -> ()  [unwired: 1 out]
            n555 = property on="自动控制" class="Bool (严格)"("Value"=FALSE ("自动控制")) -> ()  [unwired: 2 in, 2 out]
          }
        }
      }
    }
  }
  n556 = while {
    tunnel: w1 -> [w1022]
    stop <- FALSE stop-if-true
    w1021 = FALSE ("值(信号)")
    w1023 = T29."Enabled" ("禁用")
    n557 = event shown="[0] \"Run\": 鼠标按下" {
      selector: _ -> [_]
      dyn-events: _ -> [_]
      timeout: _ -> [_]
      tunnel: w1022 -> [w1026]
      event "Run": Mouse Down {
        n558 = event-data() -> ()  [unwired: 1 in, 8 out]
        n559 = flat-sequence {
          tunnel: [w1028] -> w1027
          tunnel: w1026 -> [w1028]
          tunnel: w1027 -> [w1042]
          frame #0 {
            w1029 = FALSE
            w1030 = T29."Disabled and Grayed Out" ("禁用")
            n560 = property on="溢出？" class="Bool (严格)"("Value"=w1029) -> ()  [unwired: 2 in, 2 out]
            n561 = property on="列表框" class="LstBox (严格)"("SelColor"=u32 16722474 ("选择颜色 2")) -> ()  [unwired: 2 in, 2 out]
            n562 = property class="Clust (严格)"("DisabledEnum"=w1030) -> ()  [unwired: 2 in, 2 out]
            n563 = property on="Run" class="Bool (严格)"("DisabledEnum"=w1030) -> ()  [unwired: 2 in, 2 out]
            n564 = property class="Clust (严格)"("DisabledEnum"=w1030) -> ()  [unwired: 2 in, 2 out]
            n565 = property class="Clust (严格)"("DisabledEnum"=w1030) -> ()  [unwired: 2 in, 2 out]
            n566 = property class="Clust (严格)"("DisabledEnum"=w1030) -> ()  [unwired: 2 in, 2 out]
            "编辑列表框" <- w1029
          }
          frame #1 {
            (unwired) 1 ("队列最大值（-1，无限）")
            n567 = event shown="[0] \"Abort\": 值改变" {
              selector: _ -> [_]
              dyn-events: _ -> [_]
              timeout: _ -> [_]
              event "Abort": Value Change {
                n568 = event-data() -> ()  [unwired: 1 in, 3 out]
                n569 = property on="Aborting" class="Bool (严格)"("Value"=TRUE ("元素")) -> ()  [unwired: 2 in, 2 out]
              }
            }
            n570 = Unbundle By Name "按名称解除捆绑"(w1042) -> ("Instrument Type"=w1040:T3, "行数"=w1034:refnum<vi>)
            n571 = local write "Running"(TRUE ("running")) -> ()
            n572 = property on="列表框" class="LstBox (严格)"() -> ("Item Names"=w1048:string[])  [unwired: 2 in, 2 out]
            n573 = while {
              shift-right: [w1059] -> w1037
              shift-left: bool[] [] -> [w1058]
              tunnel: w1048 -> [w1057]
              i -> [w1056]
              stop <- w1052 stop-if-true
              n574 = Array Size(array=w1057) -> (size(s)=w1053:i32)
              n575 = flat-sequence {
                tunnel: w1056 -> [w1061]
                tunnel: [w1062] -> w1060
                frame #0 {
                  n576 = property on="列表框" class="LstBox (严格)"("Active Row"=w1061) -> ()  [unwired: 2 in, 2 out]
                }
                frame #1 {
                  n577 = property on="列表框" class="LstBox (严格)"() -> ("CellFontStrike"=w1062:bool)  [unwired: 2 in, 2 out]
                }
              }
              n578 = Add(x=w1056, y=1) -> (x+y=w1054:i32)
              n579 = Greater Or Equal?(x=w1054, y=w1053) -> (x >= y?=w1052:bool)
              n580 = Insert Into Array(array=w1058, new element=w1060) -> (w1059:bool[])  [unwired: 1 in]
            }
            n581 = property class="DigNum (严格)"(reference=w1034, "Value"=0 ("值")) -> ()  [unwired: 1 in, 2 out]
            n582 = case shown="\"9T mag\"" w1040 {
              tunnel: [w1050 w1051] -> w1041
              frame "PPMS", Default {
                w1050 = refnum<visa-resource-name> "GPIB0::10::INSTR"  # 6221 Resource
              }
              frame "9T mag" {
                w1051 = refnum<visa-resource-name> "GPIB1::10::INSTR"  # 6221 Resource
              }
            }
            n583 = Obtain Queue(name (unnamed)="data save" ("名称（未命名）"), element data type=string[] []) -> (queue out=w1047:refnum<queue>)  [unwired: 3 in, 2 out]
            n584 = Bundle By Name(cluster=T27 {"initialize"=enum."SR830", "6221"={"6221 Resource"="GPIB1::10::INSTR", "Delta status"=FALSE, "电流|RMS(A)"=0.0}, "SR830+6221"={"source"=0, "Current(A)"=0.0, "阻抗(Ohm)"=0.0, "SR830 1"=FALSE, "SR830 2"=FALSE, "SR830 3"=FALSE, "SR830 4"=FALSE, "VISA 1"="GPIB1::1::INSTR", "VISA 2"="GPIB1::2::INSTR", "VISA 3"="GPIB1::3::INSTR", "VISA 4"="GPIB1::4::INSTR", "Reserve 1"=-1, "Reserve 2"=-1, "Reserve 3"=-1, "Reserve 4"=-1, "Sensitivity 1"=-1, "Sensitivity 2"=0, "Sensitivity 3"=-1, "Sensitivity 4"=-1, "量程入 1"=0, "量程入 2"=0, "量程入 3"=0, "量程入 4"=0}, "2400"={"2400"=FALSE, "VISA"="GPIB0::9::INSTR", "Output Level (0)"=1e-05, "Compliance  Level (0.1)"=10.0}, "ch"={"ch"=[], "current"=[], "change?"=[], "holding current\nwhen change ch?"=TRUE}, "Instrument"={"325 Resource "="", "Input (0:A) 325"=0, "Heater Output (1:1) 325"=0, "340 Resource"="", "Input (0:A) 340"=0, "Loop (0: 1)"=0, "Input (0:B) 340"=0, "Loop (1: 1)"=0, "340 Status"=refnum, "Instrument Type"=enum."PPMS", "quantum design"=refnum, "semaphore 325"=refnum, "TCP master instance"=refnum, "M24C Resource"="", "4G supply"="", "Temp Status 24C"=refnum, "Temp"=refnum, "9T信号"=refnum, "limit"={"Field limit"=0.0, "Field rate limit"=0.0, "Temp limit"=0.0, "Temp low limit"=0.0, "Temp rate limit "=0.0}, "4g supply status"=refnum, "vi路径"="", "in-plane"="", "out-plane"="", "in-plane signal"=FALSE, "out-plane signal"=FALSE, "in plane 信号"=refnum, "pzt volt"=refnum, "Aborting"=refnum, "数据文件"=refnum, "warning"=refnum, "750 visa"="", "750 rotate"="", "335 Status 2"=refnum, "335 Resource "="", "Input (0:A) 335"=0, "Input (0:B) 335"=0, "Heater Output (1:1) 335"=0, "semaphore 340"=refnum, "semaphore 335"=refnum, "325 Status"=refnum, "semaphore 750"=refnum, "750 field status"=refnum, "camg 振荡状态"=refnum, "列表框"=refnum, "编辑列表框？"=refnum, "camg Rate"=refnum, "行数"=refnum}, "2614B"={"2614B chA"=FALSE, "2614B chB"=FALSE, "VISA"="GPIB1::5::INSTR"}, "33522b"={"33522b resource name"="GPIB0::16::INSTR", "零电压"=0.0, "最大电压"=150.0, "间隔"=3.0, "最小电压"=-50.0, "PZT Scan?"=FALSE}, "gating type"=enum."2614(daul)", "层数"=0, "行数"=0, "是否处理"=[]} ("config in"), "Instrument"=w1042, "6221.6221 Resource"=w1041, "是否处理"=w1037, "层数"=0, "行数"=0, "gating type"=Gating_type."null") -> (w1039:T27)
            n585 = Flush Queue(queue=w1047) -> (queue out=w1038:refnum<queue>)  [unwired: 1 in, 2 out]
            n586 = call "seq analyse.vi"("config"=w1039, "数据队列"=w1038) -> ()  [unwired: 7 in, 2 out]
            n587 = call "Save Data (SubVI).vi"("簇"=w1039, "队列输入"=w1038) -> ()  [unwired: 10 in]
          }
        }
      }
    }
    n588 = property on="Abort" class="Bool (严格)"("Value"=w1021) -> ()  [unwired: 2 in, 2 out]
    n589 = property on="Run" class="Bool (严格)"("Value"=w1021) -> ()  [unwired: 2 in, 2 out]
    n590 = property on="Aborting" class="Bool (严格)"("Value"=w1021) -> ()  [unwired: 2 in, 2 out]
    n591 = property class="Clust (严格)"("DisabledEnum"=w1023) -> ()  [unwired: 2 in, 2 out]
    n592 = property on="Run" class="Bool (严格)"("DisabledEnum"=w1023) -> ()  [unwired: 2 in, 2 out]
    n593 = property class="Clust (严格)"("DisabledEnum"=w1023) -> ()  [unwired: 2 in, 2 out]
    n594 = property class="Clust (严格)"("DisabledEnum"=w1023) -> ()  [unwired: 2 in, 2 out]
    n595 = property class="Clust (严格)"("DisabledEnum"=w1023) -> ()  [unwired: 2 in, 2 out]
    "Running" <- FALSE
  }
  n596 = while {
    stop <- FALSE stop-if-true
    n597 = event shown="[0] \"gating type\": 值改变" {
      selector: _ -> [_]
      dyn-events: _ -> [_]
      timeout: _ -> [_]
      event Value Change {
        n598 = event-data() -> ("NewVal"=w1067:T1)  [unwired: 1 in, 5 out]
        n599 = case shown="\"null\", 默认" w1067 {
          tunnel: [errorcluster {"status"=FALSE, "code"=0, "source"=""} ("错误输入（无错误）") errorcluster {"status"=FALSE, "code"=0, "source"=""} ("错误输入（无错误）") errorcluster {"status"=FALSE, "code"=0, "source"=""} ("错误输入（无错误）") errorcluster {"status"=FALSE, "code"=0, "source"=""} ("错误输入（无错误）")] -> w1065
          frame "null", Default {
          }
          frame "2614(daul)" {
          }
          frame "2400" {
          }
          frame "6517B" {
          }
        }
        n600 = property on="gating type" class="Enum (严格)"(error in=w1065, "Value"=Gating_type."null" ("gating type")) -> ()  [unwired: 1 in, 2 out]
      }
    }
  }
